vi "DAISY_slow_control_2_15.vi"() -> ()   [LabVIEW 2018]
uses:
  4623b864-5764-45c6-9cb2-3e18237880ca.vi
  fa57f61f-0bb9-49ac-92eb-fcb40add4dbb.vi
  <vilib>/DAQmx/read.llb/DAQmx Read (Analog 1D DBL NChan 1Samp).vi
  ffb0d1b3-ef19-4e2e-b36e-7277177ef4b3.vi
  9a1acc8a-69db-4048-9e4c-bb07d66d2422.vi
  <vilib>/DAQmx/create/channels.llb/DAQmx Create Channel (AI-Voltage-Basic).vi
  <vilib>/DAQmx/create/channels.llb/DAQmx Create Channel (AI-Current-Basic).vi
  <vilib>/DAQmx/create/channels.llb/DAQmx Create Channel (AI-Temperature-RTD).vi
  <vilib>/DAQmx/miscellaneous.llb/DAQmx Fill In Error Info.vi
  <vilib>/Utility/file.llb/Read Delimited Spreadsheet (string).vi
  <instrlib>/Lake Shore 335/Lake Shore 335.lvlib
  <instrlib>/CAEN PSM/CAEN PSM.lvlib
  <resource>/objmgr/daqmx.rc
panel:
  out "Heater":dbl
  out "Coldhead":dbl
  out "Cycle number":i32
  out "Alarm state":bool
  out "Timestamp last \nmeasured (UPS)":timestamp
  out "Auto-clear":bool
  in  "Auto-clear data?":bool
  in  "Clear data":bool
  in  "Clear data every N cycles":dbl=1000000.0
  in  "N samples":i32=30
  out "Average Flow (SLPM)":dbl caption="Flow (SLPM)"
  out "CAEN Ch. Names":string[](array[string])
  in  "Cycles to execute":dbl=5.0 format="%#_13g"
  out "Detector Pressure":dbl
  in  "N samples":i32=20
  in  "Allows tabs on \nfront panel":T1(tab)
  in  "Anode ch.":enum16{"1", "2", "3", "4"}(ring)=enum."3"
  in  "CAEN unit selector":enum16{"CAEN 1", "CAEN 2"}(ring)
  in  "Multipliers":dbl[](array[numeric])=[1.0, 1.0, 1.0, 1.0, 1.0, 1.0, 1.0, 1.0]
  in  "Offsets\nsubtracted":dbl[](array[numeric])=[0.0, 0.0, 0.0, 0.0, 0.0, 0.0, 0.0, 0.0]
  in  "Channel Names (9207, ai8:15)":string[](array[string])=["i0", "i1", "i2", "i3", "i4", "i5", "i6", "i7"] caption="\"Other\""
  in  "Flow meter input:":u16(ring)=3 items=["v0", "v1", "v2", "v3", "v4", "v5", "v6", "v7"]
  in  "Detector pressure input:":u16(ring) items=["v0", "v1", "v2", "v3", "v4", "v5", "v6", "v7"]
  in  "Channel Names (9207, ai0:7)":string[](array[string])=["v0", "v1", "v2", "v3", "v4", "v5", "v6", "v7"] caption="\"Other\""
  in  "Multipliers":dbl[](array[numeric])=[1.0, 1.0, 1.0, 1.0, 1.0, 1.0, 1.0, 1.0]
  in  "Offsets\nsubtracted":dbl[](array[numeric])=[0.0, 0.0, 0.0, 0.0, 0.0, 0.0, 0.0, 0.0]
  in  "Voltage channels":tag[](array[tag])=["9207/ai0", "9207/ai1", "9207/ai2", "9207/ai3", "9207/ai4", "9207/ai5", "9207/ai6", "9207/ai7"]
  in  "COM-port CAEN":refnum<visa-resource-name>
  in  "Run lakeshore?":bool
  in  "ID Query":bool
  in  "COM-port LakeShore":refnum<visa-resource-name>
  in  "PID settings":cluster{"P":dbl, "I":dbl, "D":dbl}={"P"=50.0, "I"=20.0, "D"=120.0}
  in  "Heater range":u16(ring) items=["Off", "Low (On)", "Medium", "High"]
  in  "Current channels":tag[](array[tag])=["9207/ai8", "9207/ai9", "9207/ai10", "9207/ai11", "9207/ai12", "9207/ai13", "9207/ai14", "9207/ai15"]
  in  "Channel Names (CAEN)":string[](array[string])=["PMT 1", "PMT 2", "Anode", "Cathode", "Top gate", "Bottom gate", "Other 1", "Other 2"]
  in  "RTD Type":i32(ring)=10071 items=["Pt3750"=12481, "Pt3851"=10071, "Pt3911"=12482, "Pt3916"=10069, "Pt3920"=10053, "Pt3928"=12483, "Custom"=10137]
  in  "Module 1 channels (slot 1)":tag[](array[tag])=["cDAQ2Mod2/ai0", "cDAQ2Mod2/ai1", "cDAQ2Mod2/ai2", "cDAQ2Mod2/ai3", "cDAQ2Mod2/ai4", "cDAQ2Mod2/ai5", "cDAQ2Mod2/ai6", "cDAQ2Mod2/ai7"]
  in  "Resistance Configuration":i32(ring)=3 items=["3-Wire"=3, "4-Wire"=4]
  in  "R (T = 0°C):":dbl=100.0 format="%_4g"
  in  "B":dbl
  in  "A":dbl
  in  "C":dbl
  in  "Module 2 channels (slot 2)":tag[](array[tag])=["cDAQ2Mod3/ai0", "cDAQ2Mod3/ai1", "cDAQ2Mod3/ai2", "cDAQ2Mod3/ai3", "cDAQ2Mod3/ai4", "cDAQ2Mod3/ai5", "cDAQ2Mod3/ai6", "cDAQ2Mod3/ai7"]
  in  "Shut off heater \nif Alarm is active":bool=TRUE
  in  "Re-save headers":bool
  in  "Resistance Configuration":i32(ring)=3 items=["3-Wire"=3, "4-Wire"=4]
  in  "Module 3 channels":tag[](array[tag])
  in  "RTD Type":i32(ring)=12481 items=["Pt3750"=12481, "Pt3851"=10071, "Pt3911"=12482, "Pt3916"=10069, "Pt3920"=10053, "Pt3928"=12483, "Custom"=10137]
  in  "R (T = 0°C)":dbl=1000.0 format="%0.1f"
  in  "Ignore Initialization Errors":bool=TRUE caption="Ignore init. errors?"
  out "Started up?":bool
  out "heater":i32
  in  "Setpoint (°C)":dbl=-100.0 format="%.1f"
  in  "Kill all channels":bool
  in  "Scale.Range:Minimum 8":dbl
  in  "Scale.Range:Maximum 8":dbl=4000.0
  in  "Scale.Range:Minimum 7":dbl
  in  "Scale.Range:Maximum 7":dbl=4000.0
  in  "Scale.Range:Minimum 6":dbl=-3000.0
  in  "Scale.Range:Maximum 6":dbl
  in  "Scale.Range:Minimum 5":dbl
  in  "Scale.Range:Maximum 5":dbl=3000.0
  in  "Scale.Range:Minimum 4":dbl=-5000.0
  in  "Scale.Range:Maximum 4":dbl
  in  "Scale.Range:Maximum 3":dbl=4000.0
  in  "Scale.Range:Minimum 3":dbl
  in  "Scale.Range:Maximum 2":dbl=1000.0
  in  "Scale.Range:Minimum 2":dbl
  out "CAEN 1.1":dbl(knob) scale=0.0..1000.0
  out "CAEN 1.1":string
  in  "Scale.Range:Maximum":dbl=1000.0
  in  "Scale.Range:Minimum":dbl
  out "CAEN 2.3 2":string
  out "CAEN 2.2 2":string
  out "Channel Names":string[](array[string])
  out "CAEN 2.3":dbl(knob) scale=0.0..4000.0
  out "CAEN 2.2":dbl(knob) scale=0.0..4000.0
  out "CAEN 2.1":string
  out "CAEN 2.0":string
  out "CAEN 1.3":string
  out "CAEN 1.2":string
  out "CAEN 1.0":string
  out "Channel Names":string[](array[string])
  in  "Set to zero (ramp down)":bool
  out "CAEN 2.1":dbl(knob) scale=0.0..-3000.0
  out "CAEN 2.0":dbl(knob) scale=0.0..3000.0
  in  "Apply Voltage":bool
  in  "VSet (V)":dbl[](array[numeric])
  in  "IMax (uA)":dbl[](array[numeric])
  in  "VMax (V)":dbl[](array[numeric])
  out "CAEN 1.3":dbl(knob) scale=0.0..-5000.0
  out "CAEN 1.2":dbl(knob) scale=0.0..4000.0
  out "CAEN 1.0":dbl(knob) scale=0.0..1000.0
  out "Vmon (V)":dbl[](array[numeric])
  out "IMon (uA)":dbl[](array[numeric])
  in  "Reset anode\nperiodically?":bool
  in  "Kill every Y minutes":i32=10
  in  "Keep off for X seconds":i32=10
  out "?":bool
  out "Killed":bool
  out "Restarted":bool
  out "Anode timers":timestamp[](array[timestamp])
  out "Seconds until \nanode autokill":dbl format="%.2g"
  out "Seconds until \nanode reset":dbl format="%.2g"
  in  "Temperature channel selector":u16(ring) items=["0"=0, "1"=1, "2"=2, "3"=3, "4"=4, "5"=5, "6"=6, "7"=7, "Average"=666]
  out "Heater power (%)":cluster{timestamp[], dbl[]}[](graph)
  out "Flow (SLPM)":cluster{timestamp[], dbl[]}[](graph)
  out "9207 (ai 0:7, Volts)":cluster{timestamp[], dbl[]}[](graph)
  out "Phase Diagram":cluster{"X":dbl, "Y":dbl}[](graph)
  out "Setup Temperature (9216 0:15, °C)":cluster{timestamp[], dbl[]}[](graph)
  out "LakeShore readings":dbl[](array[numeric])
  out "Low Temperature (9226 0:7 and LakeShore A;B, °C)":cluster{timestamp[], dbl[]}[](graph)
  in  "Reset?":bool
  out "Integrated Flow (SL)":dbl
  in  "Pause?":bool
  in  "\"Sound\" alarm":bool
  in  "Sound alarm\nFrequency (Hz)":dbl=1260.0
  in  "Send status email now":bool
  out "Email error":i32
  out "source":string
  in  "Number of Bonus lines":i32=1
  out "Names (optional)":string[](array[string])
  in  "Send daily email?":bool=TRUE
  in  "Phone numbers":string[](array[string])
  out "Alarm (or test) message":string
  in  "Alarm\nMaster switch":bool
  in  "Repeat Alarm SMS\nevery N minutes":dbl=15.0
  in  "Test alarm":bool
  out "Warning":bool
  in  "UPS":bool
  in  "UPS Voltage \nLower Threshold":dbl=220.0
  out "NI mod 2&3 status":bool
  in  "NI mod 2&3":bool
  in  "NI mod 1":bool
  in  "CAEN 2":bool
  in  "CAEN 1":bool
  in  "LakeShore":bool
  out "Det. P. warning":bool
  out "Boolean 6":bool
  out "Boolean 5":bool
  out "Boolean 4":bool
  out "Boolean 3":bool
  out "Boolean 2":bool
  out "Boolean":bool
  in  "T 6":bool
  in  "T 5":bool
  in  "T 4":bool
  in  "T 3":bool
  in  "T 2":bool
  in  "T 1":bool
  in  "Detector Pressure":bool
  in  "Overpressure threshold":dbl
  in  "Underpressure threshold":dbl
  out "Comm. status":bool
  in  "High Temp threshold":dbl format="%#_13g"
  in  "Low Temp threshold":dbl format="%#_13g"
  out "LakeShore status":bool
  out "NI mod1 (P) status":bool
  out "CAEN 1 status":bool
  out "CAEN 2 status":bool
  out "Initialization status":bool
  out "Minimum input voltage measured":dbl
  out "Alarm active 2":bool
  out "SMS error":string
  out "Status email preview":string
  in  "Send status email at time:":string="14:00"
  in  "Email Addresses":string[](array[string])
  in  "return address":string="xamsups@gmail.com"
  out "NI 9226":errorcluster
  in  "HV Channel status":string="Click the button to request the latest High Voltage channel status.\nView another channel with the arrows, or typing 0 through 3."
  out "CAEN 1":T2(array[cluster])
  out "CAEN 2":T2(array[cluster])
  in  "Query HV status":bool
  in  "LabVIEW error code":string="Google this"
  in  "String 7":string="A checkmark means \"No error\" and false. A red X means an error occurred"
  out "\"status\"":bool
  in  "\"source\"":string="This may show two things: the latest executed VI in the task chain, in reverse order, or: which VI produced an error, with a short description. If the error can't easily be resolved, google the code."
  out "NI 9216 x2":errorcluster
  out "CAEN 1":errorcluster
  out "CAEN 2":errorcluster
  out "Lakeshore":errorcluster
  out "NI 9207":errorcluster
  out "Temp A":dbl
  out "Temp B":dbl
  in  "Temperature Channel Selector":u16(ring) items=["0", "1", "2", "3", "4", "5", "6", "7"]
  out "Historical Large Phase Diagram":cluster{dbl[], dbl[]}[](graph)
  out "Large Phase Diagram":cluster{"X":dbl, "Y":dbl}[](graph)
  in  "Temperature Channel Selector":u16(ring) items=["0"=0, "1"=1, "2"=2, "3"=3, "4"=4, "5"=5, "6"=6, "7"=7, "Average"=666]
  out "PT1000 data":dbl[](array[numeric]) format="%0.2f"
  out "9207 (V; A) Converted":dbl[](array[numeric])
  out "9216 #1 (°C)":dbl[](array[numeric])
  out "9216 #2 (°C)":dbl[](array[numeric])
  out "Raw readouts (V, mA)":dbl[](array[numeric]) format="%0.2f"
  out "Det.P input #":i32
  out "Flow input #":i32
  out "PT100 data":dbl[](array[numeric]) format="%0.2f"
  out "9207 (ai 8:15, Amperes)":cluster{timestamp[], dbl[]}[](graph)
  in  "Kill voltage":bool
  in  "stop":bool
  out "Voltages":dbl[](array[numeric])
  out "TOBA appended":dbl[][](array[numeric])
  in  "Read T every N cycles":i32=2
  out "Time until next cycle":dbl format="%.3g"
  in  "Time per cycle (s)":i32=2 caption="Time Target (s)"
  # "<- Proof of concept for New/Old T + New P"
  # "Remove ^this^ array, just for testing and takes up lots of resources"
  # "Moving averages"
  # "CAEN settings"
  # "NI 9216 Temperature settings"
  # "NI 9207 Voltage settings"
  # "NI 9207 Current settings"
  # "If RTD type is custom,\nspecify the Callendar-\nVan Dusen parameters"
  # "Anode connected to:"
  # "Channel:"
  # "Lakeshore settings"
  # "NI 9226 Temperature settings"
  # "Miscellaneous"
  # "Gain (P) (XX.X)"
  # "Reset (I) (XX.X)"
  # "Rate (D) (X.X%)"
  # "Data"
  # "Scale:"
  # "to"
  # "to"
  # "Scale:"
  # "Time of last reset"
  # "Time of last reactivation"
  # "to"
  # "Scale:"
  # "to"
  # "Scale:"
  # "Settings"
  # "Scale:"
  # "to"
  # "Scale:"
  # "to"
  # "Scale:"
  # "to"
  # "to"
  # "Scale:"
  # "ADD LAKESHORE TEMPS"
  # "Alarm indicators and arms"
  # "Detector Thresholds"
  # "Daily status email"
  # "SMS and sound alarm"
  # "Alarm conditions"
  # "Temperature channels:"
  # "Uninterruptable Power Supply"
  # "Task information"
  # "High Voltage channel status"
  # "Error info example"
  # "Channel"
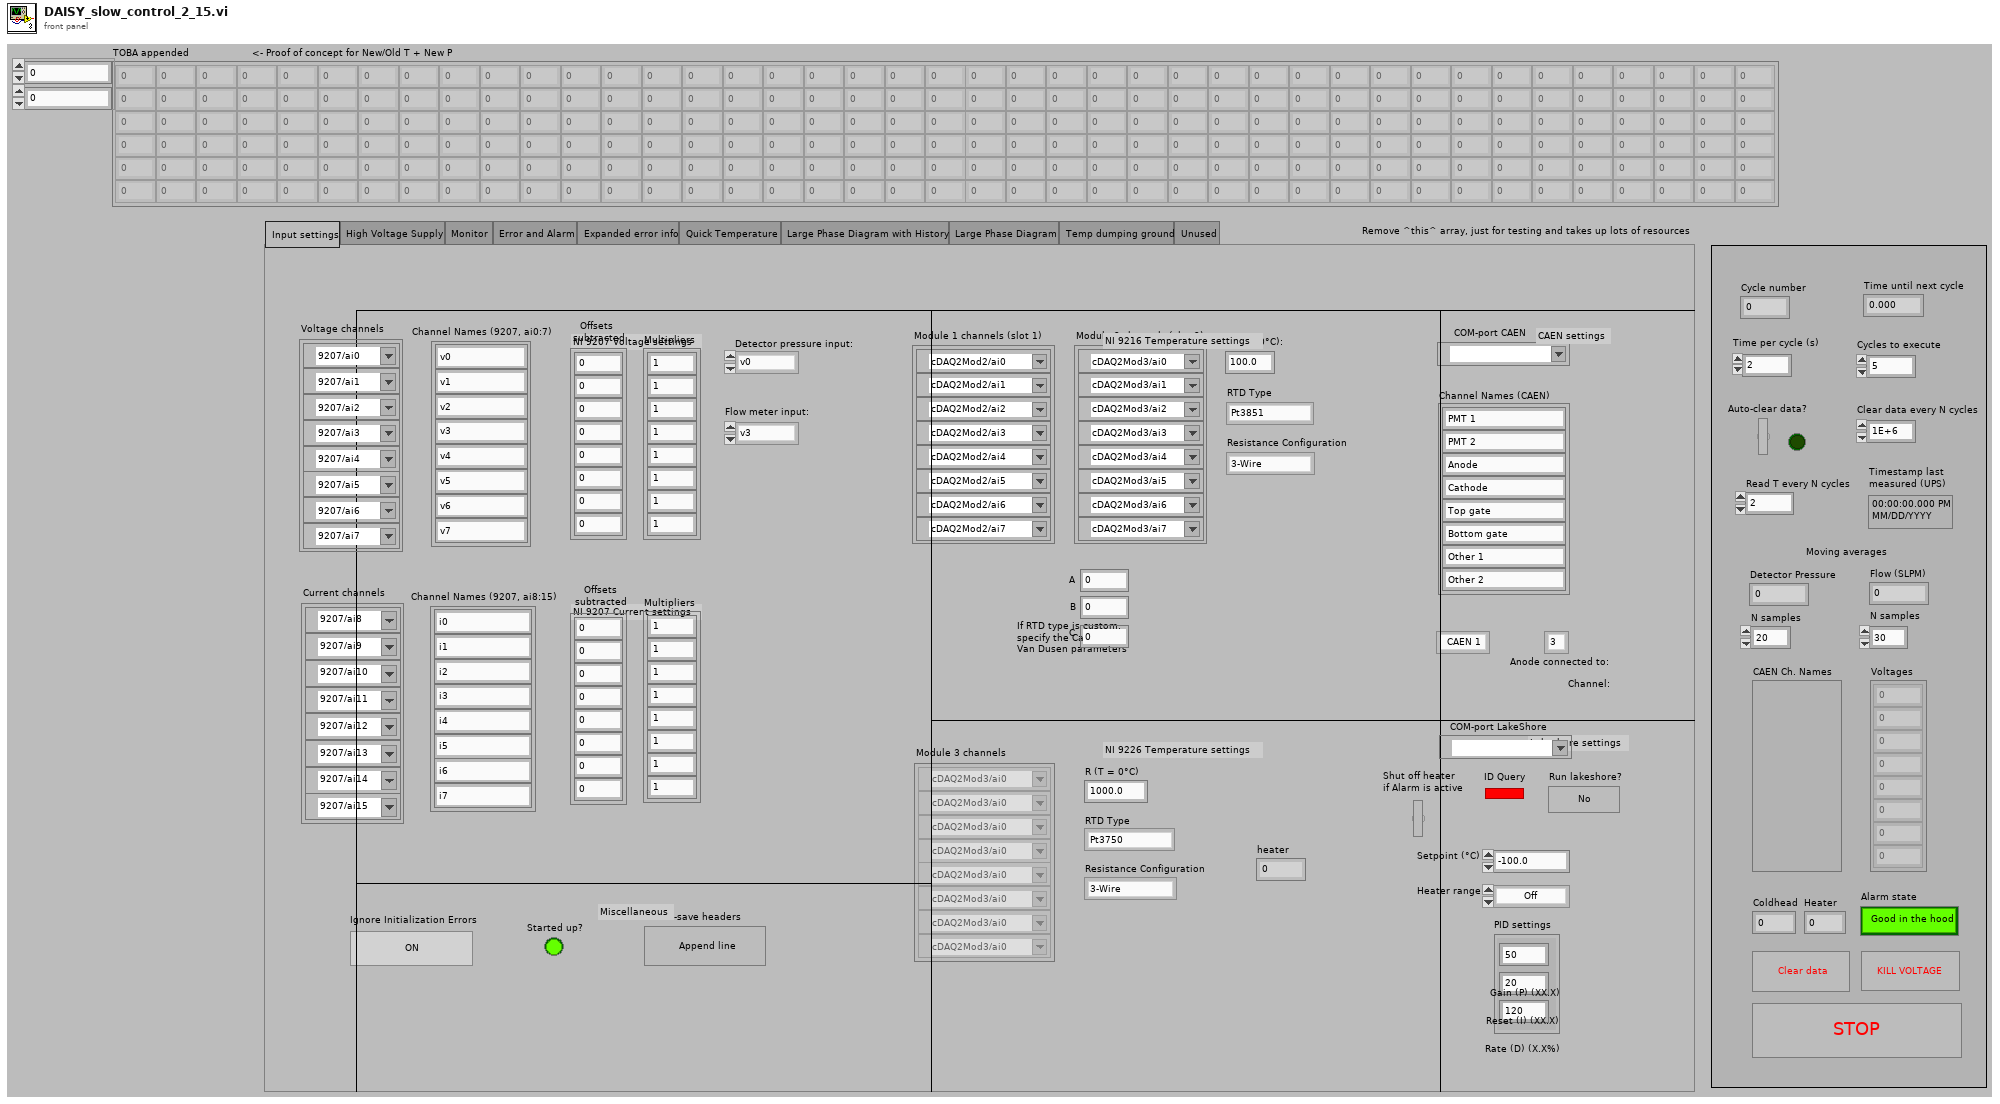
[diagram p1: front panel]
types:
  T1 = enum32{"Input settings", "High Voltage Supply", "Monitor", "Error and Alarm", "Expanded error info", "Quick Temperature", "Large Phase Diagram with History", "Large Phase Diagram", "Temp dumping ground", "Unused"}
  T2 = cluster{"ON":bool, "RUP":bool, "RDW":bool, "OVC":bool, "OVV":bool, "UNV":bool, "MAXV":bool, "TRIP":bool, "OVP":bool, "OVT":bool, "DIS":bool, "KILL":bool, "ILK":bool, "NOCAL":bool}[]
  T3 = cluster{"Baud Rate":u32, "Parity":u16, "Data Bits":u16, "Stop Bits":u16, "Flow Control":u16}
  T4 = typedef "CAEN PSM.lvlib/BoardHandle.ctl" = cluster{"VISA resource name":refnum<visa-resource-name>, "Board address":u8, "NChannels":u8}
  T5 = cluster{"task out":refnum<k21>, "error out":errorcluster}
  T6 = cluster{"VISA resource name out":refnum<visa-resource-name>, "error out":errorcluster}
  T7 = cluster{"VISA resource name":refnum<visa-resource-name>, "Board address":u8, "NChannels":u8}[]
  T8 = cluster{"VISA resource name":refnum<visa-resource-name>, "Board address":u8, "NChannels":u8}
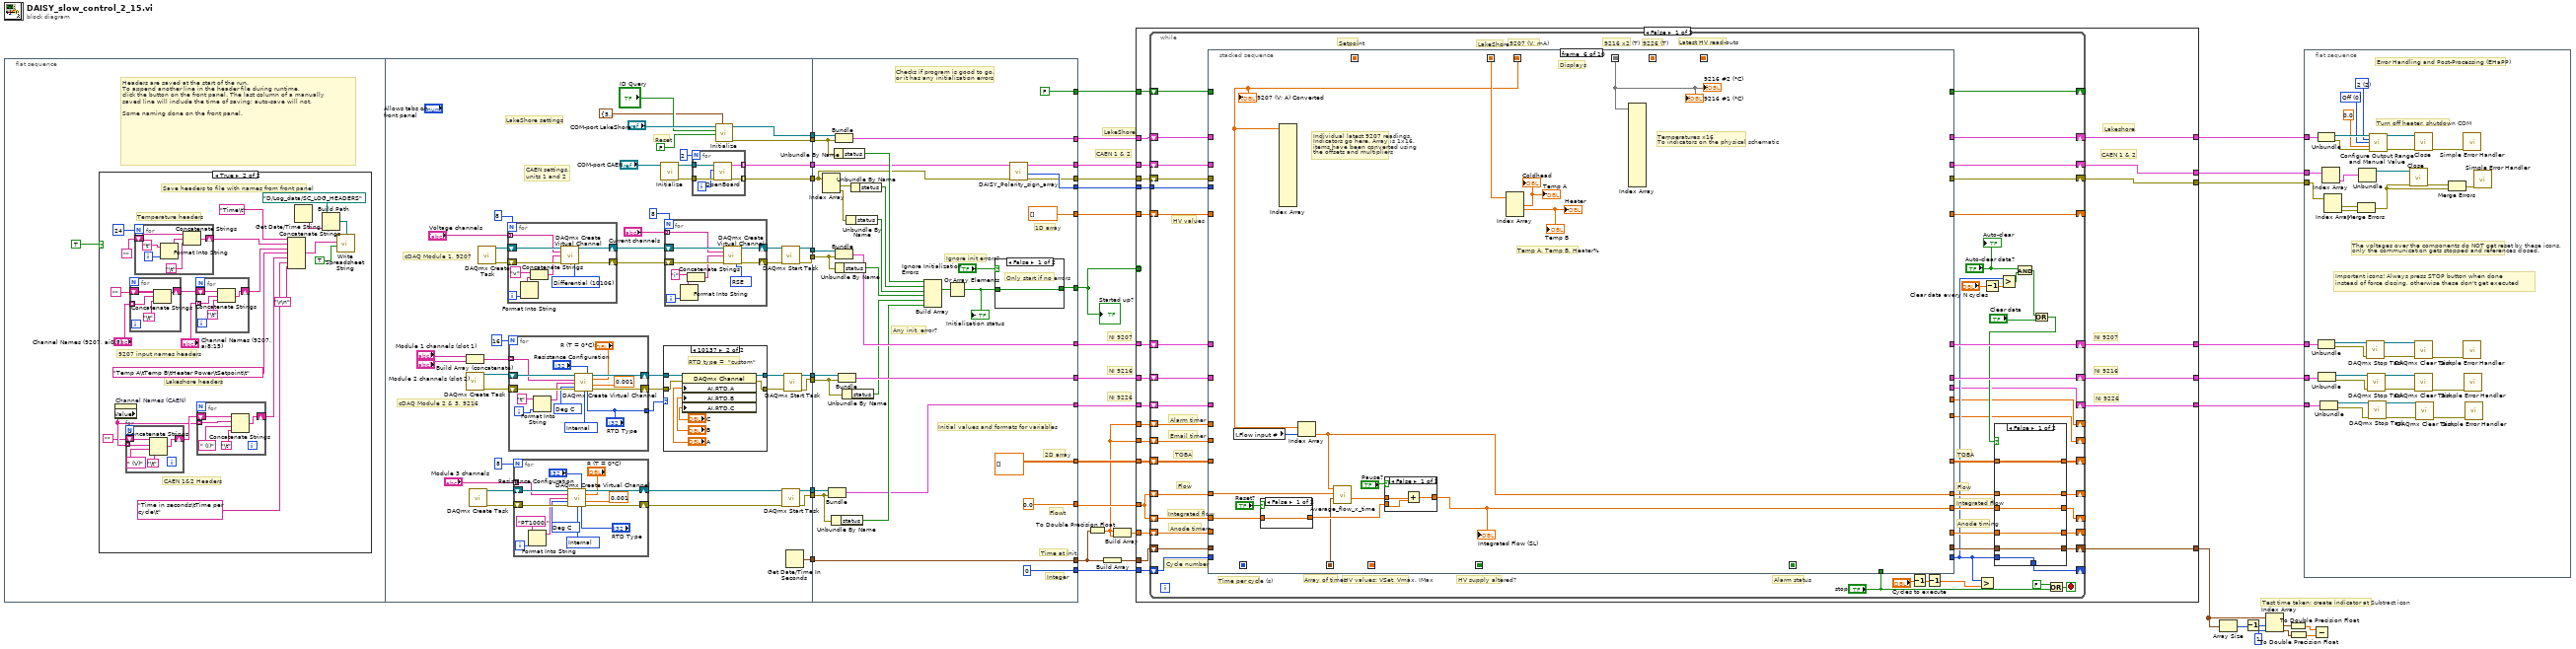
[diagram p0: block diagram]
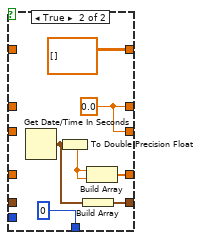
[diagram p2: hidden frame]
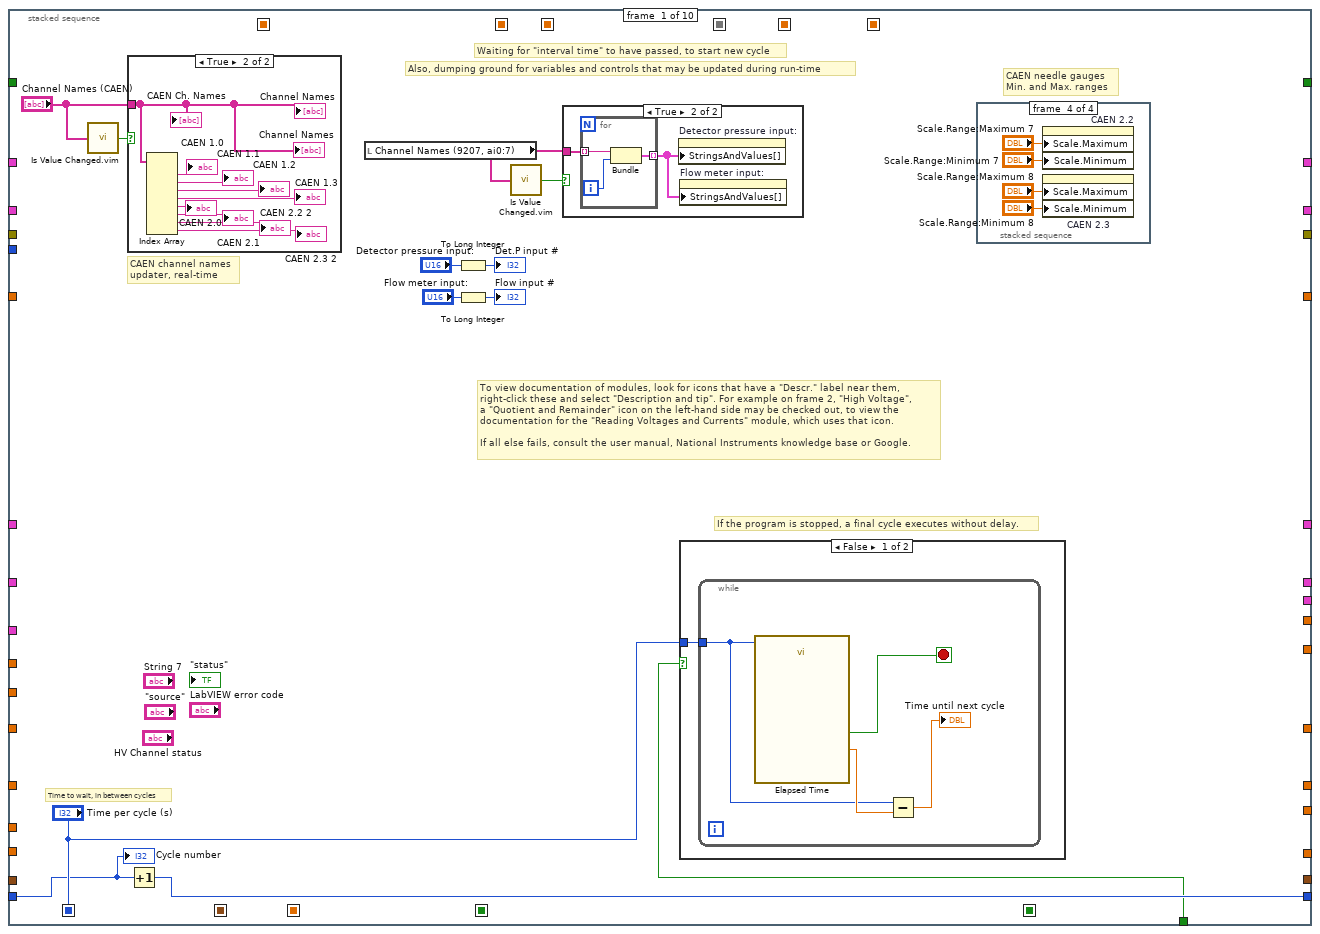
[diagram p3: hidden frame]
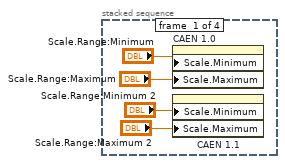
[diagram p6: hidden frame]
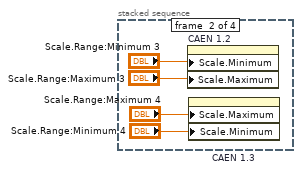
[diagram p7: hidden frame]
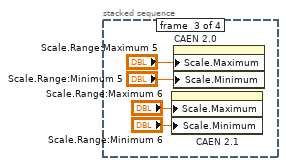
[diagram p8: hidden frame]
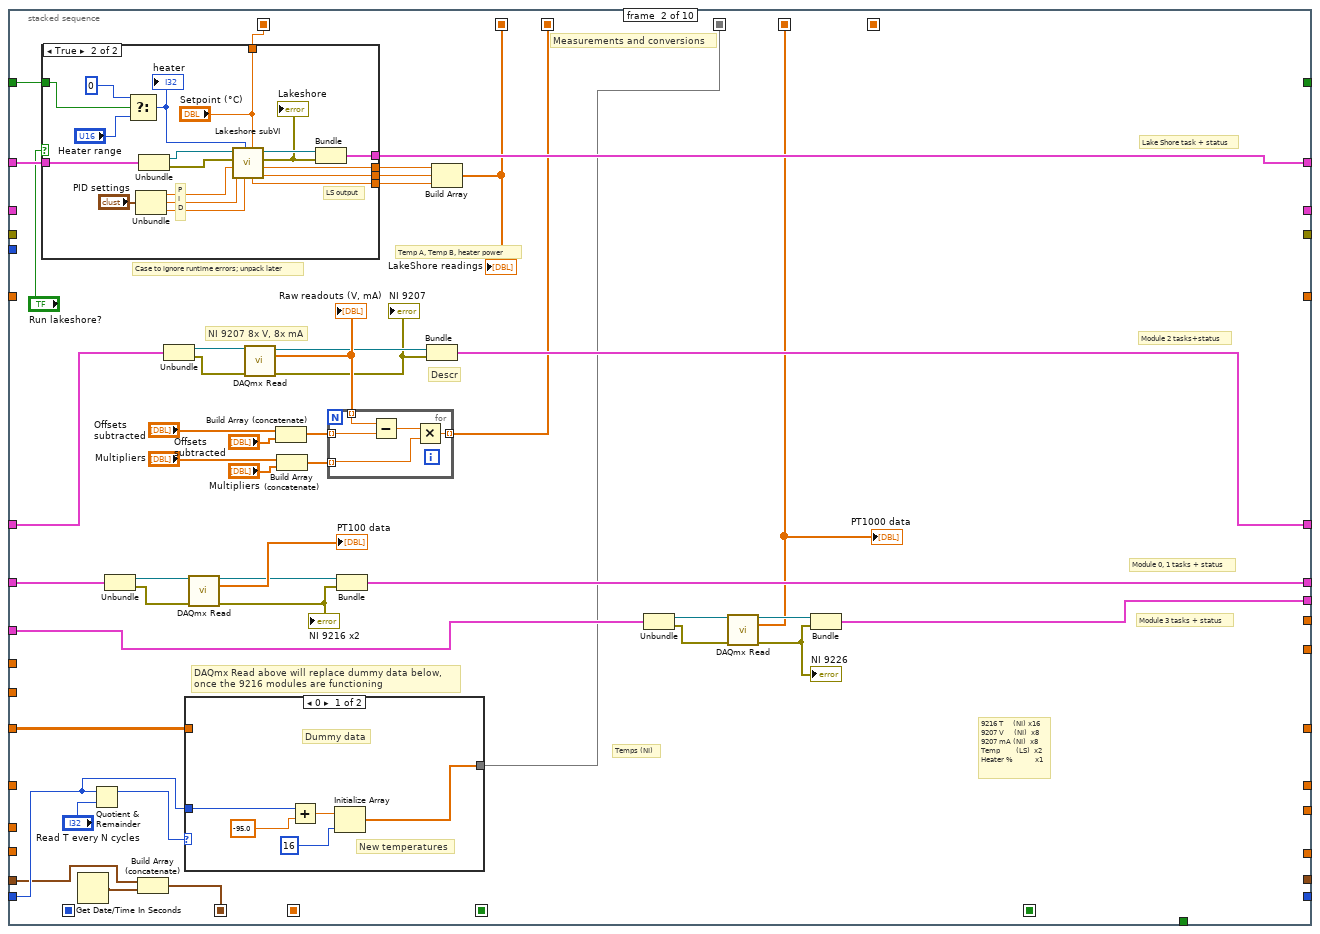
[diagram p10: hidden frame]
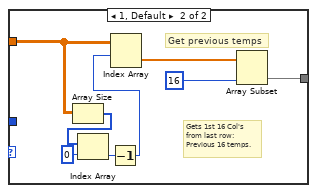
[diagram p11: hidden frame]
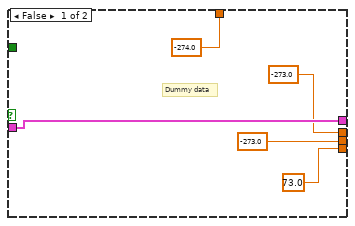
[diagram p12: hidden frame]
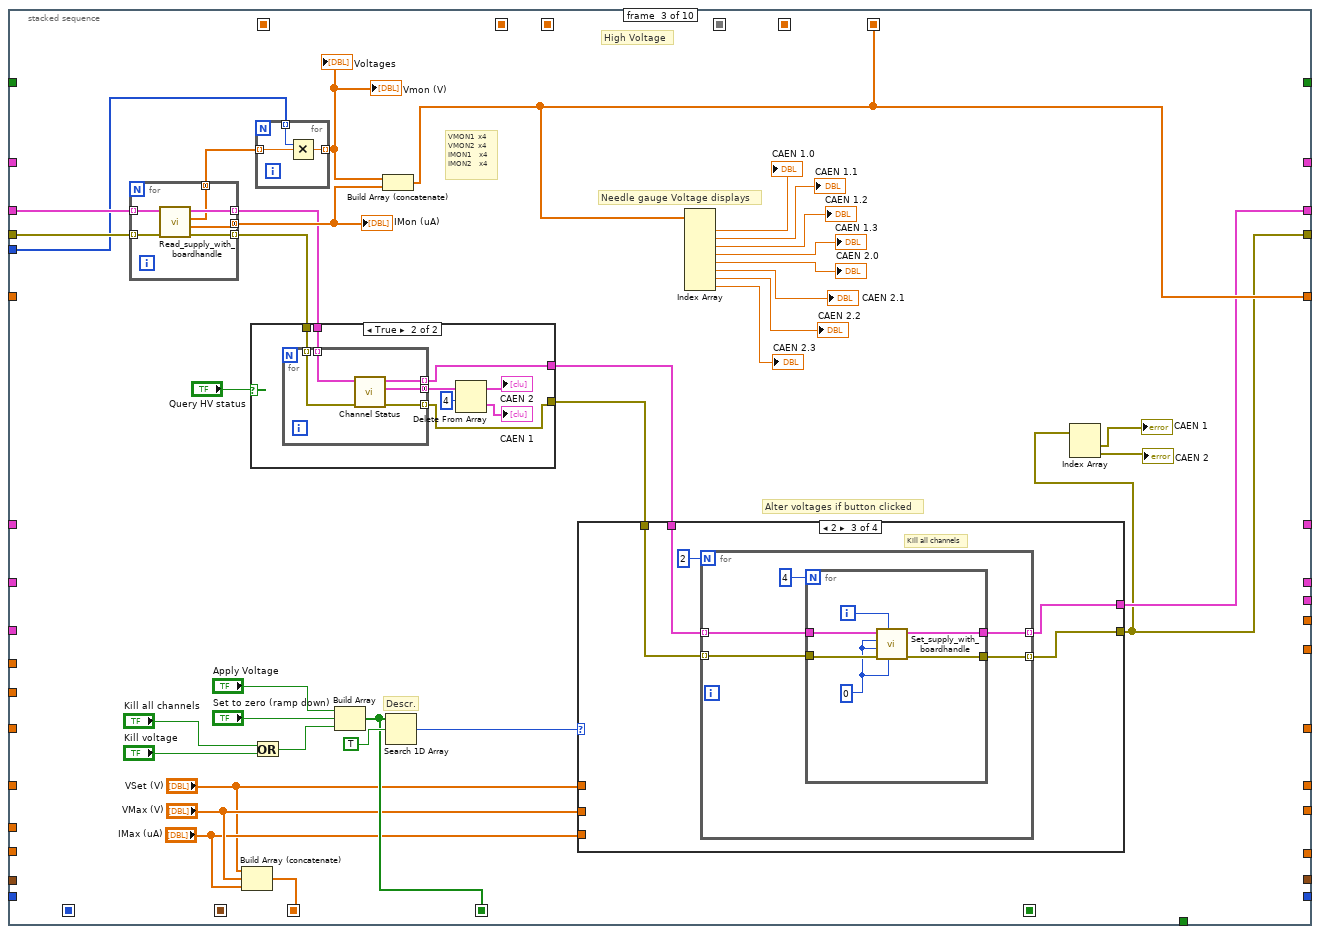
[diagram p13: hidden frame]
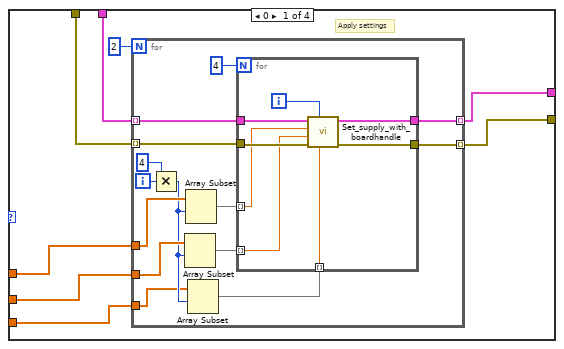
[diagram p14: hidden frame]
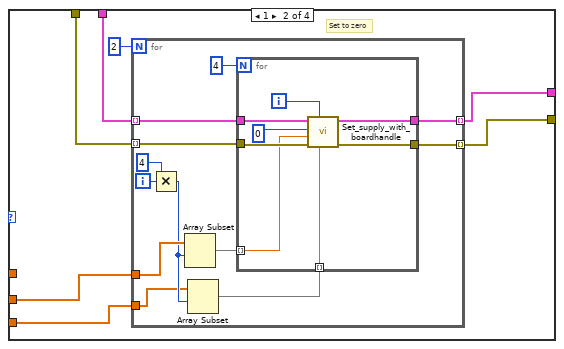
[diagram p15: hidden frame]
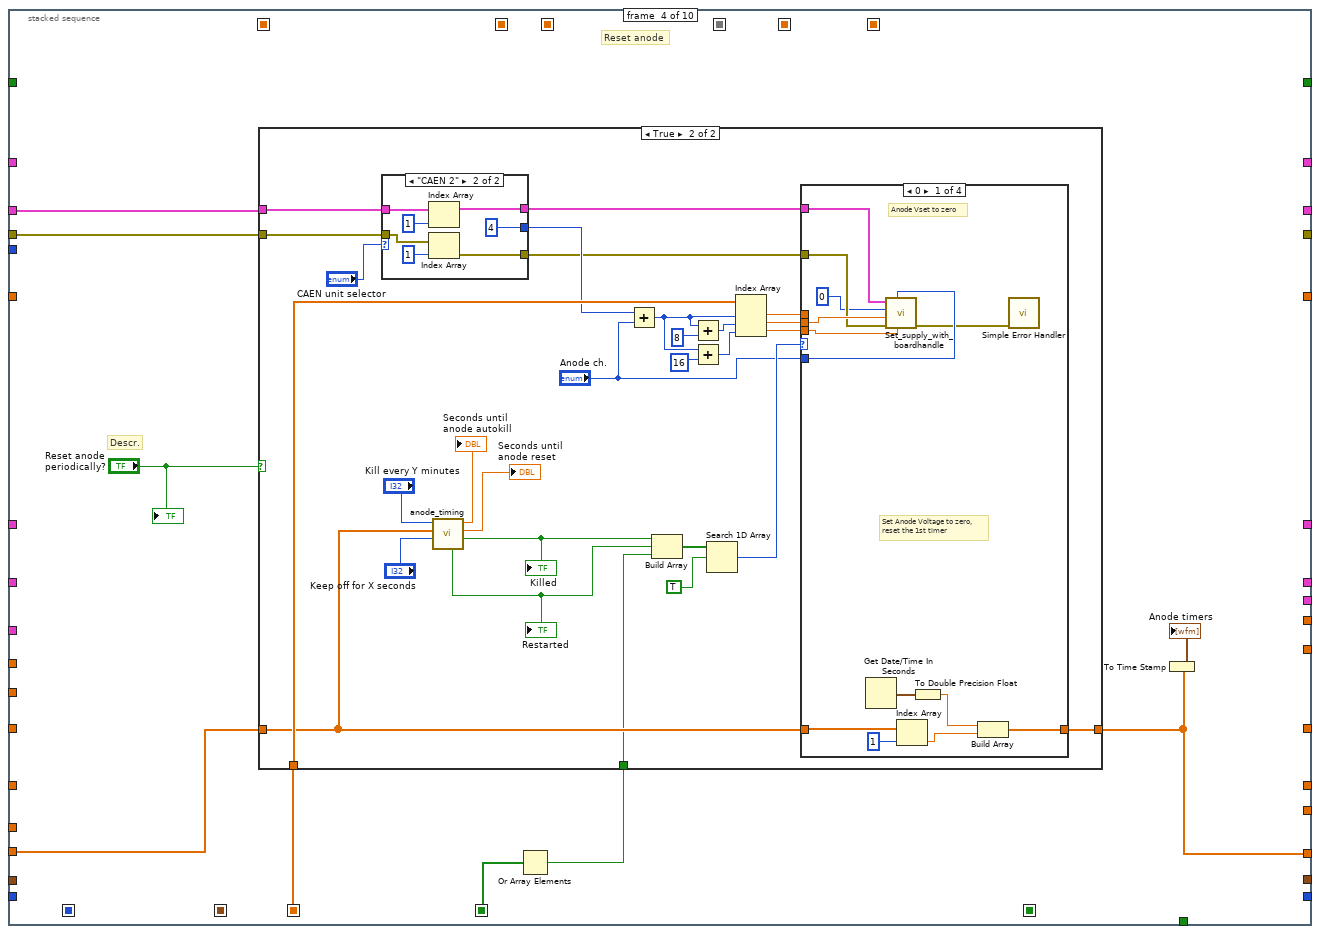
[diagram p18: hidden frame]
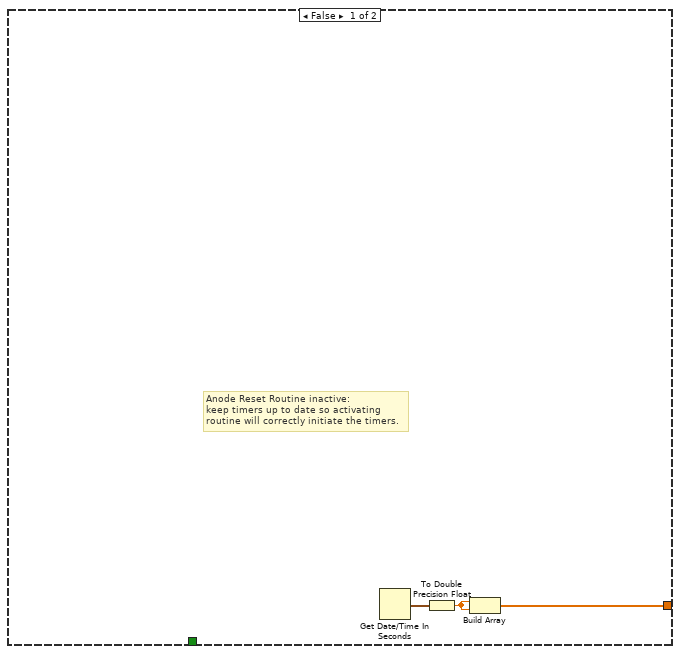
[diagram p19: hidden frame]
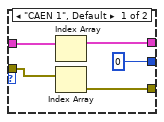
[diagram p20: hidden frame]
diagram:
  # "NI 9226"
  # "NI 9216"
  # "Test time taken: create indicator at Subtract icon"
  # "NI 9207"
  # "CAEN 1 & 2"
  # "LakeShore"
  n1 = flat-sequence {
    tunnel: [w131] -> w42
    tunnel: [w130] -> w41
    tunnel: [w127] -> w40
    tunnel: [w115] -> w39
    tunnel: [w126] -> w35
    tunnel: [w116] -> w21
    tunnel: [w110] -> w14
    tunnel: [w109] -> w13
    tunnel: [w95] -> w9
    tunnel: [w94] -> w8
    tunnel: [w90] -> w4
    tunnel: w42 -> [w228]
    tunnel: w41 -> [w227]
    tunnel: w40 -> [w200]
    tunnel: w39 -> [w220]
    tunnel: [w229] -> w27
    tunnel: [0.0] -> w26
    tunnel: [dbl[] []] -> w38
    tunnel: [dbl[][] []] -> w15
    tunnel: [0] -> w37
    tunnel: [w226] -> w36
    tunnel: [w225] -> w25
    tunnel: w35 -> [w225]
    tunnel: [FALSE] -> w22
    tunnel: w21 -> [w221]
    tunnel: [w219] -> w20
    tunnel: w14 -> [w212]
    tunnel: w13 -> [w211]
    tunnel: [w210] -> w12
    tunnel: w9 -> [w207]
    tunnel: w8 -> [w206]
    tunnel: [w204] -> w7
    tunnel: [w199] -> w5
    tunnel: w4 -> [w201]
    tunnel: [w198] -> w3
    tunnel: [w197] -> w2
    frame #0 {
      # "Headers are saved at the start of the run.\nTo append another line in the header file during runtime,\nclick the button on the front panel. The last column of a manually\nsaved line will include the time of saving; auto-save will not.\n\nSome naming done on the front panel."
      n2 = case shown="True" TRUE {
        frame False {
        }
        frame True {
          # "CAEN 1&2 Headers"
          # "Lakeshore headers"
          # "9207 input names headers"
          # "Temperature headers"
          # "Save headers to file with names from front panel"
          n3 = property on="Channel Names (CAEN)" class="Arr (strict)"() -> ("Value"=w49:string[])  [unwired: 2 in, 2 out]
          n4 = for {
            tunnel: w49 -> [w73] mode=indexing
            shift-right: [w71] -> w50
            shift-left: "" -> [w70]
            n5 = Concatenate Strings(w70, w73, " (V)", "\t") -> (w71:string)
          }
          n6 = for {
            shift-right: [w81] -> w53
            shift-left: "" -> [w82]
            tunnel: "Channel Names (9207, ai0:7)" -> [w79] mode=indexing
            n7 = Concatenate Strings(w82, w79, "\t") -> (w81:string)
          }
          n8 = for {
            N: 24 -> [_]
            shift-right: [w83] -> w56
            shift-left: "" -> [w84]
            i -> [w88]
            n9 = Format Into String(initial string="t", w88) -> (resulting string=w86:string)  [unwired: 2 in, 1 out]
            n10 = Concatenate Strings(w84, w86, "\t") -> (w83:string)
          }
          n11 = for {
            shift-right: [w76] -> w52
            shift-left: w53 -> [w78]
            tunnel: "Channel Names (9207, ai8:15)" -> [w75] mode=indexing
            n12 = Concatenate Strings(w78, w75, "\t") -> (w76:string)
          }
          n13 = for {
            shift-right: [w66] -> w48
            shift-left: w50 -> [w67]
            tunnel: w49 -> [w65] mode=indexing
            n14 = Concatenate Strings(w67, w65, " (I)", "\t") -> (w66:string)
          }
          n15 = Concatenate Strings("Time\t", w56, w52, "Temp A\tTemp B\tHeater Power\tSetpoint\t", w48, "Time in seconds\tTime per cycle\t", "\r\n") -> (w55:string)
          n16 = Get Date/Time String() -> (date string=w59:string)  [unwired: 3 in, 1 out]
          n17 = Build Path(base path=path "D:/Log_data/SC_LOG_HEADERS" ("file path (dialog if empty)"), name or relative path=w59) -> (appended path=w60:path)
          n18 = call <vilib>:"Write Spreadsheet String.vi"("append to file? (new file:F)"=TRUE, "spreadsheet string"=w55, "file path (dialog if empty)"=w60) -> ()  [unwired: 7 in, 2 out]
        }
      }
    }
    frame #1 {
      # "cDAQ Module 2 & 3, 9216"
      # "cDAQ Module 1, 9207"
      # "CAEN settings,\nunits 1 and 2"
      # "Reset"
      # "LakeShore settings"
      n19 = call <vilib>:"DAQmx Create Task.vi"() -> ("task out"=w92:refnum<k21>, "error out"=w111:errorcluster)  [unwired: 14 in]
      n20 = Build Array (concatenate)("Module 1 channels (slot 1)", "Module 2 channels (slot 2)") -> (w106:tag[])
      n21 = call <vilib>:"DAQmx Create Task.vi"() -> ("task out"=w100:refnum<k21>, "error out"=w99:errorcluster)  [unwired: 14 in]
      n22 = call <vilib>:"DAQmx Create Task.vi"() -> ("task out"=w123:refnum<k21>, "error out"=w122:errorcluster)  [unwired: 14 in]
      n23 = for {
        N: 8 -> [_]
        shift-right: [w192] -> w120
        shift-left: w123 -> [w191]
        shift-right: [w193] -> w119
        shift-left: w122 -> [w189]
        tunnel: "Voltage channels" -> [w190] mode=indexing
        i -> [w195]
        w187 = 10106 items=["Default"=-1, "RSE"=10083, "NRSE"=10078, "Differential"=10106, "Pseudodifferential"=12529] ("input terminal configuration")
        n24 = Format Into String(w195) -> (resulting string=w194:string)  [unwired: 3 in, 1 out]
        n25 = Concatenate Strings("v" ("string"), w194) -> (w188:string)
        n26 = call-poly <vilib>:"DAQmx Create Virtual Channel.vi"("task in"=w191, "input terminal configuration"=w187, "physical channels"=w190, "name to assign"=w188, "error in"=w189) -> ("task out"=w192:refnum<k21>, "error out"=w193:errorcluster)  [unwired: 9 in]
      }
      n27 = for {
        N: 16 -> [_]
        shift-right: [w173] -> w91
        shift-left: w92 -> [w176]
        shift-right: [w174] -> w105
        shift-left: w111 -> [w175]
        tunnel: w106 -> [w172] mode=indexing
        tunnel: ["RTD Type"] -> w102
        i -> [w170]
        w168 = 10200 items=["Internal"=10200, "External"=10167, "None"=10230] ("Current Excitation Source")
        w167 = 10143 items=["Deg C"=10143, "Deg F"=10144, "Kelvins"=10325, "Deg R"=10145, "From Custom Scale"=10065] ("units")
        n28 = Format Into String(initial string="t", w170) -> (resulting string=w169:string)  [unwired: 2 in, 1 out]
        n29 = call-poly <vilib>:"DAQmx Create Virtual Channel.vi"("task in"=w176, "resistance configuration"="Resistance Configuration", "physical channels"=w172, "r0"="R (T = 0°C):", "name to assign"=w169, "units"=w167, "current excitation value"=0.001, "error in"=w175, "current excitation source"=w168, "rtd type"="RTD Type") -> ("task out"=w173:refnum<k21>, "error out"=w174:errorcluster)  [unwired: 4 in]
      }
      n30 = for {
        N: 8 -> [_]
        shift-right: [w151] -> w97
        shift-left: w100 -> [w150]
        shift-right: [w152] -> w96
        shift-left: w99 -> [w153]
        tunnel: "Module 3 channels" -> [w148] mode=indexing
        i -> [w146]
        w142 = 10200 items=["Internal"=10200, "External"=10167, "None"=10230] ("current excitation source")
        w144 = 10143 items=["Deg C"=10143, "Deg F"=10144, "Kelvins"=10325, "Deg R"=10145, "From Custom Scale"=10065] ("units")
        n31 = Format Into String(initial string="PT1000.", w146) -> (resulting string=w145:string)  [unwired: 2 in, 1 out]
        n32 = call-poly <vilib>:"DAQmx Create Virtual Channel.vi"("task in"=w150, "resistance configuration"="Resistance Configuration", "physical channels"=w148, "r0"="R (T = 0°C)", "name to assign"=w145, "units"=w144, "current excitation value"=0.001, "error in"=w153, "current excitation source"=w142, "rtd type"="RTD Type") -> ("task out"=w151:refnum<k21>, "error out"=w152:errorcluster)  [unwired: 4 in]
      }
      n33 = call <instrlib>:"Initialize.vi"("VISA resource name"="COM-port CAEN") -> ("error out"=w128:errorcluster, "VISA resource name out"=w124:refnum<visa-resource-name>)  [unwired: 9 in]
      n34 = case shown="10137" w102 {
        tunnel: w91 -> [w155 w159]
        tunnel: w105 -> [w154 w158]
        tunnel: [w155 w157] -> w104
        tunnel: [w154 w156] -> w103
        frame 0, Default {
          # "Don't need to specify the A, B, C\nvalues if RTD type is not \"custom\""
        }
        frame 10137 {
          # "RTD type =  \"custom\""
          n35 = property class="DAQmx Channel"(reference=w159, error in=w158, "AI.RTD.A"="A", "AI.RTD.B"="B", "AI.RTD.C"="C") -> (reference out=w157:refnum<k21>, error out=w156:errorcluster)
        }
      }
      n36 = for {
        N: 8 -> [_]
        shift-right: [w178] -> w117
        shift-left: w120 -> [w185]
        shift-right: [w177] -> w118
        shift-left: w119 -> [w184]
        tunnel: "Current channels" -> [w183] mode=indexing
        i -> [w182]
        w186 = 10083 items=["default"=-1, "RSE"=10083, "NRSE"=10078, "Differential"=10106, "Pseudodifferential"=12529] ("input terminal configuration")
        n37 = Format Into String(w182) -> (resulting string=w180:string)  [unwired: 3 in, 1 out]
        n38 = Concatenate Strings("i", w180) -> (w179:string)
        n39 = call-poly <vilib>:"DAQmx Create Virtual Channel.vi"("task in"=w185, "input terminal configuration"=w186, "physical channels"=w183, "name to assign"=w179, "error in"=w184) -> ("task out"=w178:refnum<k21>, "error out"=w177:errorcluster)  [unwired: 9 in]
      }
      n40 = for {
        N: 2 -> [_]
        tunnel: w124 -> [w137]
        tunnel: [w135] -> w90 mode=indexing
        tunnel: w128 -> [w139]
        tunnel: [w138] -> w127 mode=indexing
        i -> [w136]
        n41 = call <instrlib>:"OpenBoard.vi"("error in (no error)"=w139, "Board Address"=w136, "VISA resource name"=w137) -> ("error out"=w138:errorcluster, "BoardHandle"=w135:T4)  [unwired: 7 in]
      }
      n42 = call <instrlib>:"Initialize.vi"("Serial Configuration"=T3 {"Baud Rate"=57600, "Parity"=1, "Data Bits"=7, "Stop Bits"=10, "Flow Control"=0}, "Reset (True)"=FALSE ("Reset (LakeShore)"), "ID Query (True)"="ID Query", "VISA resource name"="COM-port LakeShore") -> ("error out"=w130:errorcluster, "VISA resource name out"=w131:refnum<visa-resource-name>)  [unwired: 6 in]
      n43 = call <vilib>:"DAQmx Start Task.vi"("task/channels in"=w117, "error in"=w118) -> ("task out"=w116:refnum<k21>, "error out"=w115:errorcluster)  [unwired: 12 in]
      n44 = call <vilib>:"DAQmx Start Task.vi"("task/channels in"=w97, "error in"=w96) -> ("task out"=w95:refnum<k21>, "error out"=w94:errorcluster)  [unwired: 12 in]
      n45 = call <vilib>:"DAQmx Start Task.vi"("task/channels in"=w104, "error in"=w103) -> ("task out"=w110:refnum<k21>, "error out"=w109:errorcluster)  [unwired: 12 in]
      n46 = Get Date/Time In Seconds() -> (seconds since 1Jan1904=w126:timestamp)
    }
    frame #2 {
      # "1D array"
      # "Initial values and formats for variables"
      # "Time at init."
      # "Integer"
      # "2D array"
      # "Flowt"
      # "Checks if program is good to go,\nor it has any initialization errors"
      # "Ignore init errors?"
      # "Any init. error?"
      n47 = Index Array(array=w200) -> (element #1=w203:errorcluster, element #2=w202:errorcluster)  [unwired: 2 in]
      n48 = Bundle("task out"=w207, "error out"=w206) -> (w204:T5)  [unwired: 1 in]
      n49 = Unbundle By Name(w206) -> ("status"=w205:bool)
      n50 = Unbundle By Name(w227) -> ("status"=w213:bool)
      n51 = Bundle("VISA resource name out"=w228, "error out"=w227) -> (w226:T6)  [unwired: 1 in]
      n52 = Unbundle By Name(w220) -> ("status"=w214:bool)
      n53 = Bundle("task out"=w221, "error out"=w220) -> (w219:T5)  [unwired: 1 in]
      n54 = Bundle("task out"=w212, "error out"=w211) -> (w210:T5)  [unwired: 1 in]
      n55 = Unbundle By Name(w211) -> ("status"=w209:bool)
      n56 = Unbundle By Name(w202) -> ("status"=w224:bool)
      n57 = Unbundle By Name(w203) -> ("status"=w230:bool)
      n58 = Build Array(w213, w230, w214, w224, w209, w205) -> (w231:bool[])
      n59 = Or Array Elements(Boolean array=w231) -> (logical OR=w208:bool)
      "Initialization status" <- w208
      n60 = case shown="False" "Ignore Initialization Errors" {
        tunnel: [w232 FALSE] -> w229
        tunnel: w208 -> [w232 _]
        frame False {
          # "Only start if no errors"
        }
        frame True {
          # "Always start program"
        }
      }
      n61 = call "DAISY_Polarity_sign_array.vi"("error in (no error)"=w200, "BoardHandles"=w201) -> ("Errors Out"=w197:errorcluster[], "Polarity signs"=w199:i32[], "Board Handles Out"=w198:T7)  [unwired: 7 in]
    }
  }
  n62 = To Double Precision Float(number=w25) -> (double precision float=w10:dbl)
  n63 = Build Array(w25) -> (w34:timestamp[])
  n64 = Build Array(w10, w10) -> (w24:dbl[])
  n65 = case shown="False" w27 {
    selector: w27 -> [_ w1106]
    tunnel: [_ w1106] -> _
    tunnel: w38 -> [w251 _]
    tunnel: w37 -> [w256 _]
    tunnel: w15 -> [w255 _]
    tunnel: w36 -> [w252 w1104]
    tunnel: w34 -> [w254 _]
    tunnel: [w253 timestamp[] []] -> w30
    tunnel: w26 -> [w247 _]
    tunnel: w24 -> [w250 _]
    tunnel: [w249 w1104] -> w23
    tunnel: w22 -> [w248 _]
    tunnel: w20 -> [w246 w1103]
    tunnel: [w245 w1100] -> w19
    tunnel: [w244 w1103] -> w18
    tunnel: w12 -> [w243 w1102]
    tunnel: [w242 w1102] -> w11
    tunnel: w10 -> [w241 _]
    tunnel: w10 -> [w240 _]
    tunnel: w7 -> [w239 w1101]
    tunnel: [w238 w1101] -> w6
    tunnel: w5 -> [w237 _]
    tunnel: w3 -> [w236 w1100]
    tunnel: w2 -> [w235 w1099]
    tunnel: [w234 w1099] -> w1
    frame False {
      # "NI 9226"
      # "NI 9216"
      # "NI 9207"
      # "CAEN 1 & 2"
      # "Lakeshore"
      n66 = while {
        shift-right: [w272] -> _
        shift-left: w256 -> [w308]
        shift-right: [w285] -> _
        shift-left: w255 -> [w299]
        shift-right: [w277] -> w253
        shift-left: w254 -> [w305]
        shift-right: [w300] -> w245
        shift-left: w236 -> [w294]
        shift-right: [w302] -> _
        shift-left: w251 -> [w304]
        shift-right: [w301] -> w249
        shift-left: w252 -> [w303]
        shift-right: [w281] -> _
        shift-left: w247 -> [w296]
        shift-right: [w283] -> _
        shift-left: w247 -> [w297]
        shift-right: [w279] -> _
        shift-left: w250 -> [w295]
        shift-right: [w267] -> _
        shift-left: w248 -> [w293]
        shift-right: [w291] -> w244
        shift-left: w246 -> [w292]
        shift-right: [w289] -> w242
        shift-left: w243 -> [w290]
        shift-right: [w265] -> _
        shift-left: w241 -> [w266]
        shift-right: [w262] -> _
        shift-left: w240 -> [w263]
        shift-right: [w260] -> w238
        shift-left: w239 -> [w261]
        tunnel: w237 -> [w259]
        shift-right: [w257] -> w234
        shift-left: w235 -> [w258]
        stop <- w306 stop-if-true
        # "9226 (T)"
        # "Email timer"
        # "Alarm timer"
        # "Alarm status"
        # "LakeShore"
        # "9216 x2 (T)"
        # "9207 (V, mA)"
        # "HV supply altered?"
        # "Setpoint"
        # "Anode timing"
        # "Anode timers"
        # "Integrated flow"
        # "Flow"
        # "Flow"
        # "Integrated Flow"
        # "TOBA"
        # "Array of times"
        # "Latest HV read-outs"
        # "Time per cycle (s)"
        # "Cycle number"
        # "HV values: VSet, Vmax, IMax"
        # "HV values"
        # "TOBA"
        n67 = stacked-sequence {
          seq-local: [_ _ w484 _ _ _ _ _ _ _] -> [_ _ _ w596 _ _ _ _ _ _]
          seq-local: ["Time per cycle (s)" _ _ _ _ _ _ _ _ _] -> [_ _ _ _ _ _ w805 _ _ _]
          seq-local: [_ _ w468 _ _ _ _ _ _ _] -> [_ _ _ _ _ _ w803 _ _ _]
          seq-local: [_ w409 _ _ _ _ _ _ _ _] -> [_ _ _ _ w669 w788 _ _ _ _]
          seq-local: [_ _ w480 _ _ _ _ _ _ _] -> [_ _ _ w592 _ _ _ _ _ _]
          seq-local: [_ w402 _ _ _ _ _ _ _ _] -> [_ _ _ _ _ _ w802 _ _ _]
          seq-local: [_ w397 _ _ _ _ _ _ _ _] -> [_ _ _ _ w691 w780 w800 w912 w942 w1028]
          seq-local: [_ w371 _ _ _ _ _ _ _ _] -> [_ _ _ _ w694 w783 w807 _ _ _]
          seq-local: [_ w385 _ _ _ _ _ _ _ _] -> [_ _ _ _ w693 w782 w801 _ _ _]
          seq-local: [_ _ _ _ _ _ _ w872 _ _] -> [_ _ _ _ _ _ _ _ w944 w1029]
          seq-local: [_ w372 _ _ _ _ _ _ _ _] -> [_ _ _ _ w680 _ w799 w870 w938 w1011]
          tunnel: [w333 _ _ _ _ _ _ _ _ _] -> w271
          tunnel: "stop" -> [w332 _ _ _ _ _ _ _ _ _]
          tunnel: w308 -> [w322 w398 _ _ _ _ _ _ _ _]
          tunnel: w299 -> [_ w399 _ _ w723 _ _ _ _ _]
          tunnel: [_ _ _ _ w678 _ _ _ _ _] -> w286
          tunnel: w305 -> [_ w378 _ _ _ _ _ _ _ _]
          tunnel: w294 -> [_ _ w474 w597 _ _ _ _ _ _]
          tunnel: w304 -> [_ _ _ _ _ _ _ _ _ _]
          tunnel: w303 -> [_ w411 _ _ _ _ _ w926 _ _]
          tunnel: [_ w412 _ _ _ _ _ _ _ _] -> w301
          tunnel: [_ _ w468 _ _ _ _ _ _ _] -> w302
          tunnel: [_ _ w461 _ _ _ _ _ _ _] -> w300
          tunnel: [_ _ _ _ w669 _ _ _ _ _] -> w278
          tunnel: w296 -> [_ _ _ _ _ w786 _ _ _ _]
          tunnel: w297 -> [_ _ _ _ _ w787 _ _ _ _]
          tunnel: w295 -> [_ _ _ w598 _ _ _ _ _ _]
          tunnel: [_ _ _ w593 _ _ _ _ _ _] -> w280
          tunnel: w293 -> [_ w405 _ _ _ _ _ _ _ _]
          tunnel: w292 -> [_ w404 _ _ _ _ _ w925 _ _]
          tunnel: [_ w400 _ _ _ _ _ _ _ _] -> w291
          tunnel: [_ _ _ _ _ w785 _ _ _ _] -> w282
          tunnel: [_ _ _ _ _ w784 _ _ _ _] -> w284
          tunnel: w290 -> [_ w384 _ _ _ _ _ w913 _ _]
          tunnel: [_ w380 _ _ _ _ _ _ _ _] -> w289
          tunnel: [_ _ _ _ _ _ _ _ w946 _] -> w267
          tunnel: w266 -> [_ _ _ _ _ _ _ _ w941 _]
          tunnel: [_ _ _ _ _ _ _ _ w939 _] -> w265
          tunnel: w263 -> [_ _ _ _ _ _ _ _ _ w1016]
          tunnel: [_ _ _ _ _ _ _ _ _ w1015] -> w262
          tunnel: w261 -> [_ w377 _ _ _ _ _ _ _ _]
          tunnel: [_ w373 _ _ _ _ _ _ _ _] -> w260
          tunnel: w259 -> [_ _ w471 _ _ _ _ _ _ _]
          tunnel: w258 -> [_ _ w473 w590 _ _ _ w869 _ _]
          tunnel: [_ _ w457 _ _ _ _ _ _ _] -> w257
          frame #0 {
            # "CAEN channel names\nupdater, real-time"
            # "Also, dumping ground for variables and controls that may be updated during run-time"
            # "CAEN needle gauges\nMin. and Max. ranges"
            # "To view documentation of modules, look for icons that have a \"Descr.\" label near them,\nright-click these and select \"Description and tip\". For example on frame 2, \"High Voltage\",\na \"Quotient and Remainder\" icon on the left-hand side may be checked out, to view the\ndocumentation for the \"Reading Voltages and Currents\" module, which uses that icon. \n\nIf all else fails, consult the user manual, National Instruments knowledge base or Google."
            # "Time to wait, in between cycles"
            # "If the program is stopped, a final cycle executes without delay."
            # "Waiting for \"interval time\" to have passed, to start new cycle"
            n68 = call "Is Value Changed.vim"("value"="Channel Names (CAEN)") -> ("changed or first call?"=w325:bool)
            n69 = case shown="True" w325 {
              tunnel: "Channel Names (CAEN)" -> [_ w339]
              frame False {
              }
              frame True {
                n70 = Index Array(array=w339) -> (element #1=→"CAEN 1.0":string, element #2=→"CAEN 1.1":string, element #3=→"CAEN 1.2":string, element #4=→"CAEN 1.3":string, element #5=→"CAEN 2.0":string, element #6=→"CAEN 2.1":string, element #7=→"CAEN 2.2 2":string, element #8=→"CAEN 2.3 2":string)  [unwired: 8 in]
                "CAEN Ch. Names" <- w339
                "Channel Names" <- w339
                "Channel Names" <- w339
              }
            }
            n71 = Increment(x=w322) -> (x+1=w333:i32)
            n72 = local read "Channel Names (9207, ai0:7)"() -> (w323:string[])
            n73 = To Long Integer(number="Detector pressure input:") -> (32bit integer=→"Det.P input #":i32)
            n74 = To Long Integer(number="Flow meter input:") -> (32bit integer=→"Flow input #":i32)
            n75 = call "Is Value Changed.vim"("value"=w323) -> ("changed or first call?"=w324:bool)
            n76 = case shown="True" w324 {
              tunnel: w323 -> [_ w335]
              frame False {
                # ":D"
              }
              frame True {
                n77 = for {
                  tunnel: w335 -> [w338] mode=indexing
                  tunnel: [w336] -> w334 mode=indexing
                  i -> [w337]
                  n78 = Bundle("Or give name if \"Other\""=w338, w337) -> (w336:cluster{"Or give name if \"Other\"":string, i32})  [unwired: 1 in]
                }
                n79 = property on="Detector pressure input:" class="Ring (strict)"("StringsAndValues[]"=w334) -> ()  [unwired: 2 in, 2 out]
                n80 = property on="Flow meter input:" class="Ring (strict)"("StringsAndValues[]"=w334) -> ()  [unwired: 2 in, 2 out]
              }
            }
            n81 = case shown="False" w332 {
              tunnel: "Time per cycle (s)" -> [w364 _]
              frame False {
                n82 = while {
                  tunnel: w364 -> [w366]
                  stop <- w368 stop-if-true
                  n83 = call "Elapsed Time"("Time Target (s)"=w366) -> ("Elapsed Time (s)"=w367:dbl, "Time has Elapsed"=w368:bool)  [unwired: 11 in, 6 out]
                  n84 = Subtract(x=w366, y=w367) -> (x-y=→"Time until next cycle":dbl)
                }
              }
              frame True {
              }
            }
            n85 = stacked-sequence {
              frame #0 {
                n86 = property on="CAEN 1.0" class="Knob (strict)"("Scale.Minimum"="Scale.Range:Minimum", "Scale.Maximum"="Scale.Range:Maximum") -> ()  [unwired: 2 in, 2 out]
                n87 = property on="CAEN 1.1" class="Knob (strict)"("Scale.Minimum"="Scale.Range:Minimum 2", "Scale.Maximum"="Scale.Range:Maximum 2") -> ()  [unwired: 2 in, 2 out]
              }
              frame #1 {
                n88 = property on="CAEN 1.2" class="Knob (strict)"("Scale.Minimum"="Scale.Range:Minimum 3", "Scale.Maximum"="Scale.Range:Maximum 3") -> ()  [unwired: 2 in, 2 out]
                n89 = property on="CAEN 1.3" class="Knob (strict)"("Scale.Maximum"="Scale.Range:Maximum 4", "Scale.Minimum"="Scale.Range:Minimum 4") -> ()  [unwired: 2 in, 2 out]
              }
              frame #2 {
                n90 = property on="CAEN 2.1" class="Knob (strict)"("Scale.Maximum"="Scale.Range:Maximum 6", "Scale.Minimum"="Scale.Range:Minimum 6") -> ()  [unwired: 2 in, 2 out]
                n91 = property on="CAEN 2.0" class="Knob (strict)"("Scale.Maximum"="Scale.Range:Maximum 5", "Scale.Minimum"="Scale.Range:Minimum 5") -> ()  [unwired: 2 in, 2 out]
              }
              frame #3 {
                n92 = property on="CAEN 2.2" class="Knob (strict)"("Scale.Maximum"="Scale.Range:Maximum 7", "Scale.Minimum"="Scale.Range:Minimum 7") -> ()  [unwired: 2 in, 2 out]
                n93 = property on="CAEN 2.3" class="Knob (strict)"("Scale.Maximum"="Scale.Range:Maximum 8", "Scale.Minimum"="Scale.Range:Minimum 8") -> ()  [unwired: 2 in, 2 out]
              }
            }
            "Cycle number" <- w322
          }
          frame #1 {
            # "Module 3 tasks + status"
            # "Module 0, 1 tasks + status"
            # "Lake Shore task + status"
            # "DAQmx Read above will replace dummy data below,\nonce the 9216 modules are functioning"
            # "Descr"
            # "NI 9207 8x V, 8x mA"
            # "Case to ignore runtime errors; unpack later"
            # "Module 2 tasks+status"
            # "Temps (NI)"
            # "9216 T     (NI) x16\n9207 V     (NI)  x8\n9207 mA (NI)  x8\nTemp        (LS)  x2\nHeater %           x1"
            # "Temp A, Temp B, heater power"
            # "Measurements and conversions"
            n94 = case shown="True" "Run lakeshore?" {
              tunnel: [w435 w446] -> w412
              tunnel: w411 -> [w435 w445]
              tunnel: [-273.0 ("Input A") w444] -> w408
              tunnel: [-273.0 ("Input B") w443] -> w407
              tunnel: [73.0 ("Heater 1 (%)") w442] -> w406
              tunnel: w405 -> [_ w440]
              tunnel: [-274.0 "Setpoint (°C)"] -> w402
              frame False {
                # "Dummy data"
              }
              frame True {
                # "LS output"
                # "P\nI\nD"
                n95 = Select(t=0, s=w440, f="Heater range") -> (s? t:f=w437:i32)
                "heater" <- w437
                n96 = Unbundle("PID settings") -> ("P"=w451:dbl, "I"=w450:dbl, "D"=w449:dbl)
                n97 = Unbundle(w445) -> ("VISA resource name out"=w453:refnum<visa-resource-name>, "error out"=w452:errorcluster)
                n98 = call "Lakeshore subVI.vi"("Setpoint"="Setpoint (°C)", "Rate (D) (X.X %)"=w449, "Range"=w437, "Reset (I) (XX.X)"=w450, "Gain (P) (XX.X)"=w451, "error in (no error)"=w452, "VISA resource name"=w453) -> ("Input B"=w443:dbl, "Input A"=w444:dbl, "error out"=w447:errorcluster, "VISA resource name out"=w448:refnum<visa-resource-name>, "Heater 1 (%)"=w442:dbl)
                "Lakeshore" <- w447
                n99 = Bundle("VISA resource name out"=w448, "error out"=w447) -> (w446:T6)  [unwired: 1 in]
              }
            }
            n100 = Get Date/Time In Seconds() -> (seconds since 1Jan1904=w410:timestamp)
            n101 = Quotient & Remainder(x=w398, y="Read T every N cycles") -> (x-y*floor(x/y)=w401:i32)  [unwired: 1 out]
            n102 = Unbundle(w384) -> ("task out"=w383:refnum<k21>, "error out"=w382:errorcluster)
            n103 = Build Array (concatenate)(w378, w410) -> (w409:timestamp[])
            n104 = Unbundle(w404) -> ("task out"=w389:refnum<k21>, "error out"=w388:errorcluster)
            n105 = case shown="0" w401 {
              tunnel: w399 -> [_ w428]
              tunnel: [w421 w424] -> w371
              tunnel: w398 -> [w420 _]
              frame 0 {
                # "Dummy data"
                # "New temperatures"
                n106 = Add(x=w420, y=-95.0 ("element")) -> (x+y=w423:dbl)
                n107 = Initialize Array(w423, 16) -> (w421:dbl[])
              }
              frame 1, Default {
                # "Gets 1st 16 Col's\nfrom last row:\nPrevious 16 temps."
                # "Get previous temps"
                n108 = Array Size(array=w428) -> (size(s)=w430:i32[])
                n109 = Index Array(array=w430, index=0) -> (element=w431:i32)
                n110 = Decrement(x=w431) -> (x-1=w427:i32)
                n111 = Index Array(array=w428, index (row)=w427) -> (element=w426:dbl[])  [unwired: 1 in]
                n112 = Array Subset(array=w426, length=16) -> (w424:dbl[])  [unwired: 1 in]
              }
            }
            n113 = call-poly <vilib>:"DAQmx Read.vi"("task/channels in"=w383, "error in"=w382) -> ("task out"=w370:refnum<k21>, "data"=→"PT100 data":dbl[], "error out"=w381:errorcluster)  [unwired: 11 in]
            "NI 9216 x2" <- w381
            n114 = call-poly <vilib>:"DAQmx Read.vi"("task/channels in"=w389, "error in"=w388) -> ("task out"=w387:refnum<k21>, "data"=w396:dbl[], "error out"=w386:errorcluster)  [unwired: 11 in]
            "Raw readouts (V, mA)" <- w396
            "NI 9207" <- w386
            n115 = Build Array (concatenate)("Offsets\nsubtracted", "Offsets\nsubtracted") -> (w390:dbl[])
            n116 = Build Array (concatenate)("Multipliers", "Multipliers") -> (w393:dbl[])
            n117 = for {
              tunnel: w390 -> [w418] mode=indexing
              tunnel: w396 -> [w417] mode=indexing
              tunnel: w393 -> [w415] mode=indexing
              tunnel: [w414] -> w397 mode=indexing
              n118 = Subtract(x=w417, y=w418) -> (x-y=w416:dbl)
              n119 = Multiply(x=w416, y=w415) -> (x*y=w414:dbl)
            }
            n120 = Bundle("task out"=w370, "error out"=w381) -> (w380:T5)  [unwired: 1 in]
            n121 = Bundle("task out"=w387, "error out"=w386) -> (w400:T5)  [unwired: 1 in]
            n122 = Build Array(w408, w407, w406) -> (w385:dbl[])
            "LakeShore readings" <- w385
            n123 = Unbundle(w377) -> ("task out"=w369:refnum<k21>, "error out"=w376:errorcluster)
            n124 = call-poly <vilib>:"DAQmx Read.vi"("task/channels in"=w369, "error in"=w376) -> ("task out"=w375:refnum<k21>, "data"=w372:dbl[], "error out"=w374:errorcluster)  [unwired: 11 in]
            "NI 9226" <- w374
            "PT1000 data" <- w372
            n125 = Bundle("task out"=w375, "error out"=w374) -> (w373:T5)  [unwired: 1 in]
          }
          frame #2 {
            # "Alter voltages if button clicked"
            # "Descr."
            # "VMON1  x4 \nVMON2  x4\nIMON1    x4\nIMON2    x4"
            # "Needle gauge Voltage displays"
            # "High Voltage"
            n126 = for {
              tunnel: w474 -> [w589] mode=indexing
              tunnel: w473 -> [w588] mode=indexing
              tunnel: [w587] -> w466 mode=indexing
              tunnel: [w586] -> w465 mode=indexing
              tunnel: [w585] -> w472 mode=concatenating
              tunnel: [w584] -> w469 mode=concatenating
              n127 = call "Read_supply_with_boardhandle.vi"("error in (no error)"=w588, "BoardHandle"=w589) -> ("error out"=w586:errorcluster, "IMon values (uA)"=w584:dbl[], "VMon values (V)"=w585:dbl[], "BoardHandle out"=w587:T8)  [unwired: 6 in]
            }
            "IMon (uA)" <- w469
            n128 = Build Array (concatenate)("VSet (V)", "VMax (V)", "IMax (uA)") -> (w484:dbl[])
            n129 = case shown="True" "Query HV status" {
              tunnel: w466 -> [w567 w575]
              tunnel: w465 -> [w566 w574]
              tunnel: [w567 w569] -> w463
              tunnel: [w566 w568] -> w462
              frame False {
              }
              frame True {
                n130 = for {
                  tunnel: w575 -> [w580] mode=indexing
                  tunnel: w574 -> [w579] mode=indexing
                  tunnel: [w578] -> w569 mode=indexing
                  tunnel: [w577] -> w568 mode=indexing
                  tunnel: [w576] -> w573 mode=concatenating
                  n131 = call <instrlib>:"Channel Status.vi"("error in (no error)"=w579, "BoardHandle"=w580) -> ("error out"=w577:errorcluster, "Channel Status Array"=w576:T2, "BoardHandle out"=w578:T4)  [unwired: 7 in]
                }
                n132 = Delete From Array(array=w573, length=4) -> (deleted portion=→"CAEN 1":T2, array with subset deleted=→"CAEN 2":T2)  [unwired: 1 in]
              }
            }
            n133 = Or(x="Kill all channels", y="Kill voltage") -> (x .or. y?=w475:bool)
            n134 = for {
              tunnel: w472 -> [w582] mode=indexing
              tunnel: w471 -> [w583] mode=indexing
              tunnel: [w581] -> w470 mode=indexing
              n135 = Multiply(x=w583, y=w582) -> (x*y=w581:dbl)
            }
            "Voltages" <- w470
            "Vmon (V)" <- w470
            n136 = Build Array("Apply Voltage", "Set to zero (ramp down)", w475) -> (w480:bool[])
            n137 = Build Array (concatenate)(w470, w469) -> (w468:dbl[])
            n138 = Search 1D Array(1D array=w480, element=TRUE) -> (index of element=w464:i32)  [unwired: 1 in]
            n139 = case shown="2" w464 {
              tunnel: w463 -> [w497 w526 w551 w565]
              tunnel: w462 -> [w496 w525 w550 w564]
              tunnel: [w492 w522 w549 w565] -> w461
              tunnel: [w491 w521 w548 w564] -> w457
              tunnel: "VSet (V)" -> [w495 _ _ _]
              tunnel: "VMax (V)" -> [w494 w524 _ _]
              tunnel: "IMax (uA)" -> [w493 w523 _ _]
              frame 0 {
                # "Apply settings"
                n140 = for {
                  N: 2 -> [_]
                  tunnel: w497 -> [w511] mode=indexing
                  tunnel: w496 -> [w510] mode=indexing
                  tunnel: w495 -> [w507]
                  tunnel: w494 -> [w505]
                  tunnel: w493 -> [w503]
                  tunnel: [w500] -> w492 mode=indexing
                  tunnel: [w499] -> w491 mode=indexing
                  i -> [w509]
                  n141 = Multiply(x=4, y=w509) -> (x*y=w504:i32)
                  n142 = Array Subset(array=w505, index=w504) -> (w502:dbl[])  [unwired: 1 in]
                  n143 = Array Subset(array=w507, index=w504) -> (w506:dbl[])  [unwired: 1 in]
                  n144 = Array Subset(array=w503, index=w504) -> (w501:dbl[])  [unwired: 1 in]
                  n145 = for {
                    N: 4 -> [_]
                    tunnel: w511 -> [w519]
                    tunnel: w510 -> [w518]
                    tunnel: w506 -> [w517] mode=indexing
                    tunnel: w502 -> [w516] mode=indexing
                    tunnel: w501 -> [w515] mode=indexing
                    tunnel: [w514] -> w500
                    tunnel: [w513] -> w499
                    i -> [w520]
                    n146 = call "Set_supply_with_boardhandle.vi"("Current Limit (0.00 uA)"=w515, "Channel (0)"=w520, "error in (no error)"=w518, "Voltage Max (0.0 V)"=w516, "Voltage Level (0.0 V)"=w517, "BoardHandle"=w519) -> ("error out"=w513:errorcluster, "BoardHandle out"=w514:T8)  [unwired: 4 in]
                  }
                }
              }
              frame 1 {
                # "Set to zero"
                n147 = for {
                  N: 2 -> [_]
                  tunnel: w526 -> [w538] mode=indexing
                  tunnel: w525 -> [w537] mode=indexing
                  tunnel: w524 -> [w534]
                  tunnel: w523 -> [w532]
                  tunnel: [w529] -> w522 mode=indexing
                  tunnel: [w528] -> w521 mode=indexing
                  i -> [w536]
                  n148 = Multiply(x=4, y=w536) -> (x*y=w533:i32)
                  n149 = Array Subset(array=w534, index=w533) -> (w531:dbl[])  [unwired: 1 in]
                  n150 = Array Subset(array=w532, index=w533) -> (w530:dbl[])  [unwired: 1 in]
                  n151 = for {
                    N: 4 -> [_]
                    tunnel: w538 -> [w546]
                    tunnel: w537 -> [w545]
                    tunnel: w531 -> [w544] mode=indexing
                    tunnel: w530 -> [w543] mode=indexing
                    tunnel: [w542] -> w529
                    tunnel: [w541] -> w528
                    i -> [w547]
                    n152 = call "Set_supply_with_boardhandle.vi"("Current Limit (0.00 uA)"=w543, "Channel (0)"=w547, "error in (no error)"=w545, "Voltage Max (0.0 V)"=w544, "Voltage Level (0.0 V)"=0, "BoardHandle"=w546) -> ("error out"=w541:errorcluster, "BoardHandle out"=w542:T8)  [unwired: 4 in]
                  }
                }
              }
              frame 2 {
                # "Kill all channels"
                n153 = for {
                  N: 2 -> [_]
                  tunnel: w551 -> [w556] mode=indexing
                  tunnel: w550 -> [w555] mode=indexing
                  tunnel: [w554] -> w549 mode=indexing
                  tunnel: [w553] -> w548 mode=indexing
                  n154 = for {
                    N: 4 -> [_]
                    tunnel: w556 -> [w562]
                    tunnel: w555 -> [w561]
                    tunnel: [w560] -> w554
                    tunnel: [w559] -> w553
                    i -> [w563]
                    w558 = 0
                    n155 = call "Set_supply_with_boardhandle.vi"("Current Limit (0.00 uA)"=w558, "Channel (0)"=w563, "error in (no error)"=w561, "Voltage Max (0.0 V)"=w558, "Voltage Level (0.0 V)"=w558, "BoardHandle"=w562) -> ("error out"=w559:errorcluster, "BoardHandle out"=w560:T8)  [unwired: 4 in]
                  }
                }
              }
              frame 3, Default {
                # "Do nothing"
              }
            }
            n156 = Index Array(array=w468) -> (element #1=→"CAEN 1.0":dbl, element #2=→"CAEN 1.1":dbl, element #3=→"CAEN 1.2":dbl, element #4=→"CAEN 1.3":dbl, element #5=→"CAEN 2.0":dbl, element #6=→"CAEN 2.1":dbl, element #7=→"CAEN 2.2":dbl, element #8=→"CAEN 2.3":dbl)  [unwired: 8 in]
            n157 = Index Array(array=w457) -> (element #1=→"CAEN 1":errorcluster, element #2=→"CAEN 2":errorcluster)  [unwired: 2 in]
          }
          frame #3 {
            # "Descr."
            # "Reset anode"
            n158 = Or Array Elements(Boolean array=w592) -> (logical OR=w591:bool)
            n159 = case shown="True" "Reset anode\nperiodically?" {
              tunnel: w598 -> [_ w607]
              tunnel: w597 -> [_ w614]
              tunnel: w596 -> [_ w619]
              tunnel: w591 -> [_ w605]
              tunnel: [w599 w606] -> w593
              tunnel: w590 -> [_ w603]
              frame False {
                # "Anode Reset Routine inactive:\nkeep timers up to date so activating\nroutine will correctly initiate the timers."
                n160 = Get Date/Time In Seconds() -> (seconds since 1Jan1904=w601:timestamp)
                n161 = To Double Precision Float(number=w601) -> (double precision float=w600:dbl)
                n162 = Build Array(w600, w600) -> (w599:dbl[])
              }
              frame True {
                n163 = case shown="\"CAEN 2\"" "CAEN unit selector" {
                  tunnel: w614 -> [w634 w640]
                  tunnel: [0 4] -> w612
                  tunnel: [w632 w638] -> w604
                  tunnel: w603 -> [w631 w636]
                  tunnel: [w630 w635] -> w602
                  frame "CAEN 1", Default {
                    n164 = Index Array(array=w634) -> (element=w632:T4)  [unwired: 1 in]
                    n165 = Index Array(array=w631) -> (element=w630:errorcluster)  [unwired: 1 in]
                  }
                  frame "CAEN 2" {
                    n166 = Index Array(array=w640, index=1) -> (element=w638:T4)
                    n167 = Index Array(array=w636, index=1) -> (element=w635:errorcluster)
                  }
                }
                n168 = call "anode_timing.vi"("Keep off for X seconds"="Keep off for X seconds", "Array of timers"=w607, "Kill every Y minutes"="Kill every Y minutes") -> ("Time to kill"=w621:bool, "Time until reset"=→"Seconds until \nanode reset":dbl, "Time until autokill"=→"Seconds until \nanode autokill":dbl, "Time to reset"=w622:bool)  [unwired: 5 in]
                "Killed" <- w621
                "Restarted" <- w622
                n169 = Add(x=w612, y="Anode ch.") -> (x+y=w610:i32)
                n170 = Build Array(w621, w622, w605) -> (w625:bool[])
                n171 = Add(x=w610, y=8) -> (x+y=w615:i32)
                n172 = Add(x=w610, y=16) -> (x+y=w616:i32)
                n173 = Search 1D Array(1D array=w625, element=TRUE) -> (index of element=w624:i32)  [unwired: 1 in]
                n174 = Index Array(array=w619, index #1=w610, index #2=w615, index #3=w616) -> (element #1=w628:dbl, element #2=w626:dbl, element #3=w627:dbl)
                n175 = case shown="0" w624 {
                  tunnel: w628 -> [_ w656 _ _]
                  tunnel: w626 -> [w648 w657 _ _]
                  tunnel: w627 -> [w647 w658 _ _]
                  tunnel: "Anode ch." -> [w644 w659 _ _]
                  tunnel: w607 -> [w650 _ _ w668]
                  tunnel: [w649 w662 w665 w668] -> w606
                  tunnel: w604 -> [w645 w660 _ _]
                  tunnel: w602 -> [w646 w661 _ _]
                  frame 0 {
                    # "Set Anode Voltage to zero,\nreset the 1st timer"
                    # "Anode Vset to zero"
                    n176 = Get Date/Time In Seconds() -> (seconds since 1Jan1904=w653:timestamp)
                    n177 = call "Set_supply_with_boardhandle.vi"("Current Limit (0.00 uA)"=w647, "Channel (0)"=w644, "error in (no error)"=w646, "Voltage Max (0.0 V)"=w648, "Voltage Level (0.0 V)"=0, "BoardHandle"=w645) -> ("error out"=w643:errorcluster)  [unwired: 4 in, 1 out]
                    n178 = Index Array(array=w650, index=1) -> (element=w651:dbl)
                    n179 = To Double Precision Float(number=w653) -> (double precision float=w652:dbl)
                    n180 = Build Array(w652, w651) -> (w649:dbl[])
                    n181 = call <vilib>:"Simple Error Handler.vi"("error in (no error)"=w643) -> ()  [unwired: 4 in, 5 out]
                  }
                  frame 1 {
                    # "Set Anode Voltage to defined value,\nreset both timers"
                    # "Anode Vset applied"
                    n182 = Get Date/Time In Seconds() -> (seconds since 1Jan1904=w664:timestamp)
                    n183 = call "Set_supply_with_boardhandle.vi"("Current Limit (0.00 uA)"=w658, "Channel (0)"=w659, "error in (no error)"=w661, "Voltage Max (0.0 V)"=w657, "Voltage Level (0.0 V)"=w656, "BoardHandle"=w660) -> ("error out"=w655:errorcluster)  [unwired: 4 in, 1 out]
                    n184 = To Double Precision Float(number=w664) -> (double precision float=w663:dbl)
                    n185 = Build Array(w663, w663) -> (w662:dbl[])
                    n186 = call <vilib>:"Simple Error Handler.vi"("error in (no error)"=w655) -> ()  [unwired: 4 in, 5 out]
                  }
                  frame 2 {
                    # "Change Voltage button pressed"
                    # "Reset both timers"
                    n187 = Get Date/Time In Seconds() -> (seconds since 1Jan1904=w667:timestamp)
                    n188 = To Double Precision Float(number=w667) -> (double precision float=w666:dbl)
                    n189 = Build Array(w666, w666) -> (w665:dbl[])
                  }
                  frame 3, Default {
                    # "Timers stay at previous value,\nso difference between those and\ncurrent time keeps incrementing"
                    # "No event"
                  }
                }
              }
            }
            n190 = To Time Stamp(1:w593) -> (0:→"Anode timers":timestamp[])
            "?" <- "Reset anode\nperiodically?"
          }
          frame #4 {
            # "Det. P"
            # "Flow"
            # "Flexibly acquire indices"
            # "Plots 9207 output vs time"
            # "Descr."
            # "Moving averages"
            # "Historic graphs: Phase, 9207 ai, Flow, Heater, Temperature"
            # "Non-historic Temperature + Det. Pressure"
            # "Updated TOBA >>>"
            # "Descr."
            # "Latest Detector Pressure"
            # "Plots individual lists of Temp. vs. t"
            # "Plots and moving averages"
            n191 = Build Array (concatenate)(w694, w680, w691, w693) -> (w722:dbl[])
            n192 = Build Array (concatenate)(w723, w722) -> (w678:dbl[][])
            "TOBA appended" <- w678
            n193 = Array Size(array=w691) -> (size(s)=w690:i32)
            n194 = Array Size(array=w680) -> (size(s)=w692:i32)
            n195 = Array Size(array=w694) -> (size(s)=w681:i32)
            n196 = Add(x=w681, y=w692) -> (x+y=w676:i32)
            n197 = Add(x=w676, y=w690) -> (x+y=w689:i32)
            n198 = local read "Flow input #"() -> (w700:i32)
            n199 = local read "Det.P input #"() -> (w701:i32)
            n200 = Add(x=w689, y=2 ("disabled index (col)")) -> (x+y=w687:i32)
            n201 = Equal?(x=666, y="Temperature channel selector") -> (x = y?=w716:bool)
            n202 = Index Array(array=w678, index (col)=w687) -> (element=w686:dbl[])  [unwired: 1 in]
            n203 = case shown="True" w716 {
              tunnel: w680 -> [w761 w762]
              tunnel: [w760 w763] -> w714
              tunnel: "Temperature channel selector" -> [w759 _]
              frame False {
                n204 = Index Array(array=w761, index=w759) -> (element=w760:dbl)
              }
              frame True {
                n205 = Add Array Elements(numeric array=w762) -> (sum=w764:dbl)
                n206 = Array Size(array=w762) -> (size(s)=w765:i32)
                n207 = Divide(x=w764, y=w765) -> (x/y=w763:dbl)
              }
            }
            n208 = Add(x=w701, y=w676) -> (x+y=w710:i32)
            n209 = Add(x=w676, y=w700) -> (x+y=w708:i32)
            n210 = Bundle(w669, w686) -> (w683:cluster{timestamp[], dbl[]})  [unwired: 1 in]
            n211 = Build Array(w683) -> (→"Heater power (%)":cluster{timestamp[], dbl[]}[])
            n212 = Add(x=w681, y="Temperature Channel Selector") -> (x+y=w684:i32)
            n213 = Index Array(array=w678, index (col) #1=w710, index (col) #2=w708) -> (element #1=w709:dbl[], element #2=w698:dbl[])  [unwired: 2 in]
            n214 = local read "Det.P input #"() -> (w702:i32)
            n215 = Index Array(array=w678, index (col)=w684) -> (element=w713:dbl[])  [unwired: 1 in]
            n216 = for {
              N: 8 -> [_]
              tunnel: w678 -> [w752]
              tunnel: w669 -> [w745]
              tunnel: [w749] -> w706 mode=indexing
              tunnel: [w744] -> w705 mode=indexing
              tunnel: w676 -> [w742]
              i -> [w748]
              n217 = Add(x=w742, y=8) -> (x+y=w741:i32)
              n218 = Add(x=w742, y=w748) -> (x+y=w751:i32)
              n219 = Add(x=w748, y=w741) -> (x+y=w747:i32)
              n220 = Index Array(array=w752, index (col) #1=w751, index (col) #2=w747) -> (element #1=w750:dbl[], element #2=w746:dbl[])  [unwired: 2 in]
              n221 = Bundle(w745, w750) -> (w749:cluster{timestamp[], dbl[]})  [unwired: 1 in]
              n222 = Bundle(w745, w746) -> (w744:cluster{timestamp[], dbl[]})  [unwired: 1 in]
            }
            "9207 (ai 0:7, Volts)" <- w706
            "9207 (ai 8:15, Amperes)" <- w705
            n223 = Bundle(w713, w709) -> (w727:cluster{dbl[], dbl[]})  [unwired: 1 in]
            n224 = Index Array(array=w691, index=w702) -> (element=w728:dbl)
            n225 = call "moving_avg.vi"("N samples"="N samples", "Array"=w709) -> ("Numeric"=→"Detector Pressure":dbl)  [unwired: 9 in]
            n226 = call "moving_avg.vi"("N samples"="N samples", "Array"=w698) -> ("Numeric"=→"Average Flow (SLPM)":dbl)  [unwired: 9 in]
            n227 = Bundle(w669, w698) -> (w725:cluster{timestamp[], dbl[]})  [unwired: 1 in]
            n228 = Build Array(w727) -> (→"Historical Large Phase Diagram":cluster{dbl[], dbl[]}[])
            n229 = Bundle("Waveform"=w714, w728) -> (w732:cluster{"Waveform":dbl, dbl})  [unwired: 1 in]
            n230 = Build Array(w725) -> (→"Flow (SLPM)":cluster{timestamp[], dbl[]}[])
            n231 = Build Array(w732) -> (→"Phase Diagram":cluster{"Waveform":dbl, dbl}[])
            n232 = for {
              N: w681 -> [_]
              tunnel: w669 -> [w777]
              tunnel: [w776] -> w733 mode=indexing
              tunnel: w678 -> [w775]
              i -> [w773]
              n233 = Index Array(array=w775, index (col)=w773) -> (element=w774:dbl[])  [unwired: 1 in]
              n234 = Bundle(w777, w774) -> (w776:cluster{timestamp[], dbl[]})  [unwired: 1 in]
            }
            "Setup Temperature (9216 0:15, °C)" <- w733
            n235 = Increment(x=w676) -> (x+1=w677:i32)
            n236 = Array Size(array=w680) -> (size(s)=w679:i32)
            n237 = Equal?(x=666, y="Temperature Channel Selector") -> (x = y?=w718:bool)
            n238 = Index Array(array=w678, index (col) #1=w676, index (col) #2=w677) -> (element #1=w675:dbl[], element #2=w674:dbl[])  [unwired: 2 in]
            n239 = local read "Channel Names (9207, ai0:7)"() -> (w703:string[])
            n240 = local read "Channel Names (9207, ai8:15)"() -> (w704:string[])
            n241 = case shown="False" w718 {
              tunnel: w680 -> [w768 w769]
              tunnel: [w767 w770] -> w721
              tunnel: "Temperature Channel Selector" -> [w766 _]
              frame False {
                n242 = Index Array(array=w768, index=w766) -> (element=w767:dbl)
              }
              frame True {
                n243 = Add Array Elements(numeric array=w769) -> (sum=w771:dbl)
                n244 = Array Size(array=w769) -> (size(s)=w772:i32)
                n245 = Divide(x=w771, y=w772) -> (x/y=w770:dbl)
              }
            }
            n246 = for {
              N: w679 -> [_]
              tunnel: w669 -> [w740]
              tunnel: [w739] -> w673 mode=indexing
              tunnel: w678 -> [w738]
              tunnel: w681 -> [w734]
              i -> [w735]
              n247 = Add(x=w734, y=w735) -> (x+y=w736:i32)
              n248 = Index Array(array=w738, index (col)=w736) -> (element=w737:dbl[])  [unwired: 1 in]
              n249 = Bundle(w740, w737) -> (w739:cluster{timestamp[], dbl[]})  [unwired: 1 in]
            }
            n250 = Bundle(w669, w675) -> (w672:cluster{timestamp[], dbl[]})  [unwired: 1 in]
            n251 = Bundle(w669, w674) -> (w671:cluster{timestamp[], dbl[]})  [unwired: 1 in]
            n252 = call "Is Value Changed.vim"("value"=w704) -> ("changed or first call?"=w711:bool)
            n253 = call "Is Value Changed.vim"("value"=w703) -> ("changed or first call?"=w712:bool)
            n254 = case shown="True" w711 {
              tunnel: w704 -> [_ w753]
              frame False {
              }
              frame True {
                n255 = for {
                  tunnel: w753 -> [w754] mode=indexing
                  i -> [w755]
                  n256 = property on="9207 (ai 8:15, Amperes)" class="XYGraph (strict)"("Active Plot"=w755, "Plot.Plot Name"=w754) -> ()  [unwired: 2 in, 2 out]
                }
              }
            }
            n257 = case shown="True" w712 {
              tunnel: w703 -> [_ w756]
              frame False {
              }
              frame True {
                n258 = for {
                  tunnel: w756 -> [w757] mode=indexing
                  i -> [w758]
                  n259 = property on="9207 (ai 0:7, Volts)" class="XYGraph (strict)"("Active Plot"=w758, "Plot.Plot Name"=w757) -> ()  [unwired: 2 in, 2 out]
                }
              }
            }
            n260 = Bundle("Waveform"=w721, w728) -> (w730:cluster{"Waveform":dbl, dbl})  [unwired: 1 in]
            n261 = Build Array (concatenate)(w673, w672, w671) -> (→"Low Temperature (9226 0:7 and LakeShore A;B, °C)":cluster{timestamp[], dbl[]}[])
            n262 = Build Array(w730) -> (→"Large Phase Diagram":cluster{"Waveform":dbl, dbl}[])
          }
          frame #5 {
            # "Temp A, Temp B, Heater%"
            # "Temperatures x16\nTo indicators on the physical schematic"
            # "Individual latest 9207 readings.\nIndicators go here. Array is 1x16,\nitems have been converted using\nthe offsets and multipliers"
            # "Displays"
            n263 = local read "Flow input #"() -> (w781:i32)
            n264 = case shown="False" "Reset?" {
              tunnel: [w793 0.0] -> w789
              tunnel: w786 -> [w793 _]
              frame False {
              }
              frame True {
              }
            }
            n265 = Index Array(array=w780) -> ()  [unwired: 16 in, 16 out]
            n266 = Index Array(array=w780, index=w781) -> (element=w784:dbl)
            n267 = call "Average_flow_x_time.vi"("Array of timestamps"=w788, "Previous Flow"=w787, "Latest Flow"=w784) -> ("Volume (SL)"=w790:dbl)  [unwired: 8 in]
            n268 = case shown="False" "Pause?" {
              tunnel: w789 -> [w797 w798]
              tunnel: w790 -> [w796 _]
              tunnel: [w795 w798] -> w785
              frame False {
                n269 = Add(x=w796, y=w797) -> (x+y=w795:dbl)
              }
              frame True {
              }
            }
            "Integrated Flow (SL)" <- w785
            n270 = Index Array(array=w782) -> (element #1=→"Coldhead" →"Temp A":dbl, element #2=→"Heater" →"Temp B":dbl)  [unwired: 3 in, 1 out]
            n271 = Index Array(array=w783) -> ()  [unwired: 16 in, 16 out]
            "9207 (V; A) Converted" <- w780
            "9216 #1 (°C)" <- w783
            "9216 #2 (°C)" <- w783
          }
          frame #6 {
            # "The same order applies to the headers resaved,\nbut with an additional line, stating the date/time"
            # "-----------DATA SAVED----------\nHuman-readable timestamp  ;\nTemperatures (16),  2xNI 9216;\nTemperatures (8),        NI 9226;\nVolts, Amps  (8 x2),     NI 9207;\nTemperature (2),    Lakeshore;\nHeater power (1),  Lakeshore;\nSetpoint (1),           Lakeshore;\nHV readouts (16)          CAEN ;\nCurrent time (s)                ---   ;\nCycle time (s)                    ---   ;"
            # "Saving data"
            n272 = Get Date/Time In Seconds() -> (seconds since 1Jan1904=w821:timestamp)
            n273 = To Double Precision Float(number=w821) -> (double precision float=w804:dbl)
            n274 = Build Array (concatenate)(w807, w799, w800, w801, w802, w803, w804, w805) -> (w820:dbl[])
            n275 = Array Size(array=w807) -> (size(s)=w808:i32)
            n276 = Array Size(array=w799) -> (size(s)=w809:i32)
            n277 = Add(x=w808, y=w809) -> (x+y=w806:i32)
            n278 = Get Date/Time String() -> (date string=w814:string)  [unwired: 3 in, 1 out]
            n279 = case shown="True" "Re-save headers" {
              tunnel: w806 -> [_ w822]
              frame False {
                # "Just sit around and feel pretty"
              }
              frame True {
                w830 = ""
                # "Append line of most recent channel names to header file"
                n280 = local read "Channel Names (CAEN)"() -> (w829:string[])
                n281 = local read "Channel Names (9207, ai0:7)"() -> (w837:string[])
                n282 = for {
                  N: w822 -> [_]
                  shift-right: [w861] -> w833
                  shift-left: "" -> [w862]
                  i -> [w866]
                  n283 = Format Into String(initial string="t", w866) -> (resulting string=w864:string)  [unwired: 2 in, 1 out]
                  n284 = Concatenate Strings(w862, w864, "\t") -> (w861:string)
                }
                n285 = for {
                  shift-right: [w859] -> w835
                  shift-left: w830 -> [w860]
                  tunnel: w837 -> [w857] mode=indexing
                  n286 = Concatenate Strings(w860, w857, "\t") -> (w859:string)
                }
                n287 = local read "Channel Names (9207, ai8:15)"() -> (w836:string[])
                n288 = for {
                  tunnel: w829 -> [w851] mode=indexing
                  shift-right: [w849] -> w824
                  shift-left: w830 -> [w848]
                  n289 = Concatenate Strings(w848, w851, " (V)", "\t") -> (w849:string)
                }
                n290 = for {
                  shift-right: [w855] -> w832
                  shift-left: w835 -> [w856]
                  tunnel: w836 -> [w853] mode=indexing
                  n291 = Concatenate Strings(w856, w853, "\t") -> (w855:string)
                }
                n292 = for {
                  tunnel: w829 -> [w846] mode=indexing
                  shift-right: [w844] -> w828
                  shift-left: w824 -> [w843]
                  n293 = Concatenate Strings(w843, w846, " (I)", "\t") -> (w844:string)
                }
                n294 = Get Date/Time String() -> (date string=w841:string)  [unwired: 3 in, 1 out]
                n295 = Format Date/Time String() -> (date/time string=w823:string)  [unwired: 3 in]
                n296 = Build Path(base path=path "D:/Log_data/SC_LOG_HEADERS", name or relative path=w841) -> (appended path=w840:path)
                n297 = Concatenate Strings("Time\t", w833, w832, "Temp A\tTemp B\tHeater Power\tSetpoint\t", w828, "Time in seconds\tTime per cycle\t", w823, "\r\n") -> (w825:string)
                n298 = call <vilib>:"Write Spreadsheet String.vi"("append to file? (new file:F)"=TRUE, "spreadsheet string"=w825, "file path (dialog if empty)"=w840) -> ()  [unwired: 7 in, 2 out]
              }
            }
            n299 = Build Path(base path=path "D:/Log_data/SC_LOG", name or relative path=w814) -> (appended path=w813:path)
            n300 = Format Date/Time String() -> (date/time string=w818:string)  [unwired: 3 in]
            n301 = Array To Spreadsheet String(array=w820, 3:"%.3f" ("format string")) -> (spreadsheet string=w816:string)  [unwired: 1 in]
            n302 = Concatenate Strings(w818, "\t", w816) -> (w812:string)
            n303 = call <vilib>:"Write Spreadsheet String.vi"("append to file? (new file:F)"=TRUE, "spreadsheet string"=w812, "file path (dialog if empty)"=w813) -> ()  [unwired: 7 in, 2 out]
          }
          frame #7 {
            # "Status is True if ANY (armed)\ncondition is met"
            # "Detector P. Alert"
            # "Uninteruptable\n Power Supply Alert"
            # "Temp. Warning"
            # "Arms"
            # "Comm. Alert"
            # "Temperature Alert"
            # "Alarm conditions (Temp)"
            # "Check Alarms and Warnings"
            n304 = Index Array(array=w869) -> (element #1=w868:errorcluster, element #2=w867:errorcluster)  [unwired: 2 in]
            n305 = Unbundle By Name(w913) -> ("error out.status"=w895:bool)
            "NI mod 2&3 status" <- w895
            n306 = Unbundle By Name(w926) -> ("error out.status"=w924:bool)
            "LakeShore status" <- w924
            n307 = Unbundle By Name(w925) -> ("error out.status"=w921:bool)
            "NI mod1 (P) status" <- w921
            n308 = Unbundle By Name(w867) -> ("status"=w922:bool)
            "CAEN 2 status" <- w922
            n309 = Unbundle By Name(w868) -> ("status"=w923:bool)
            "CAEN 1 status" <- w923
            n310 = Build Array(w924, w923, w922, w921, w895) -> (w896:bool[])
            n311 = Build Array("LakeShore", "CAEN 1", "CAEN 2", "NI mod 2&3", "NI mod 1") -> (w891:bool[])
            n312 = call "check_ups.vi"() -> ("Error: no voltages read"=w875:bool, "Timestamp last measured"=→"Timestamp last \nmeasured (UPS)":timestamp, "Minimum input voltage measured"=w885:dbl)  [unwired: 8 in, 1 out]
            "Minimum input voltage measured" <- w885
            n313 = property on="Det.P input #" class="DigNum (strict)"() -> ("Value"=w911:i32)  [unwired: 2 in, 2 out]
            n314 = Or Array Elements(Boolean array=w896) -> (logical OR=→"Comm. status":bool)
            n315 = for {
              tunnel: w896 -> [w929] mode=indexing
              tunnel: w891 -> [w928] mode=indexing
              tunnel: [w927] -> w890 mode=indexing
              n316 = And(x=w929, y=w928) -> (x .and. y?=w927:bool)
            }
            n317 = Index Array(array=w912, index=w911) -> (element=w908:dbl)
            n318 = Less?(x=w885, y="UPS Voltage \nLower Threshold") -> (x < y?=w877:bool)
            n319 = Equal?(x=w885, y=-1.0) -> (x = y?=w876:bool)
            n320 = Less?(x=w908, y="Underpressure threshold") -> (x < y?=w906:bool)
            n321 = Build Array(w877, w876, w875) -> (w874:bool[])
            n322 = Or Array Elements(Boolean array=w890) -> (logical OR=w880:bool)
            n323 = Greater?(x=w908, y="Overpressure threshold") -> (0:w907:bool)
            n324 = Or(x=w907, y=w906) -> (x .or. y?=w905:bool)
            "Det. P. warning" <- w905
            n325 = Or Array Elements(Boolean array=w874) -> (logical OR=w873:bool)
            "Warning" <- w873
            n326 = And(x="UPS", y=w873) -> (x .and. y?=w879:bool)
            n327 = And(x=w905, y="Detector Pressure") -> (x .and. y?=w881:bool)
            n328 = Build Array("T 1", "T 2", "T 3", "T 4", "T 5", "T 6") -> (w871:bool[])
            n329 = for {
              tunnel: w870 -> [w930] mode=indexing
              tunnel: w871 -> [w933] mode=indexing
              tunnel: [w932] -> w882 mode=indexing
              tunnel: [w931] -> w897 mode=indexing
              n330 = Less?(x=w930, y="Low Temp threshold") -> (x < y?=w935:bool)
              n331 = Greater?(x=w930, y="High Temp threshold") -> (0:w934:bool)
              n332 = Or(x=w935, y=w934) -> (x .or. y?=w931:bool)
              n333 = And(x=w933, y=w931) -> (x .and. y?=w932:bool)
            }
            n334 = Index Array(array=w897) -> (element #1=→"Boolean":bool, element #2=→"Boolean 2":bool, element #3=→"Boolean 3":bool, element #4=→"Boolean 4":bool, element #5=→"Boolean 5":bool, element #6=→"Boolean 6":bool)  [unwired: 6 in]
            n335 = Build Array (concatenate)(w882, w881, w880, w879) -> (w878:bool[])
            n336 = Or Array Elements(Boolean array=w878) -> (logical OR=w872:bool)
            "Alarm state" <- w872
          }
          frame #8 {
            # "Testing alarm will not interfere"
            # "Act on alarm"
            n337 = Or(x="Test alarm", y=w944) -> (x .or. y?=w945:bool)
            n338 = case shown="True" w945 {
              tunnel: "Test alarm" -> [_ w952]
              tunnel: w942 -> [_ w960]
              tunnel: w938 -> [_ w959]
              tunnel: w941 -> [w948 w950]
              tunnel: "Alarm\nMaster switch" -> [_ w957]
              tunnel: [w948 w951] -> w939
              frame False {
                # "Timer stays at previous value"
              }
              frame True {
                n339 = Get Date/Time In Seconds() -> (seconds since 1Jan1904=w964:timestamp)
                n340 = case shown="True" "\"Sound\" alarm" {
                  frame False {
                  }
                  frame True {
                    n341 = call <vilib>:"Beep.vi"("use system alert? (T)"=FALSE, "duration (msec)"=u32 1000, "frequency (Hz)"="Sound alarm\nFrequency (Hz)") -> ()  [unwired: 9 in]
                  }
                }
                n342 = To Double Precision Float(number=w964) -> (double precision float=w961:dbl)
                n343 = Multiply(x="Repeat Alarm SMS\nevery N minutes", y=60.0) -> (x*y=w953:dbl)
                n344 = Subtract(x=w961, y=w950) -> (x-y=w956:dbl)
                n345 = Greater?(x=w956, y=w953) -> (0:w958:bool)
                n346 = And(x=w957, y=w958) -> (x .and. y?=w955:bool)
                n347 = Or(x=w952, y=w955) -> (x .or. y?=w954:bool)
                n348 = case shown="True" w954 {
                  tunnel: w952 -> [_ w980]
                  tunnel: w960 -> [_ w988]
                  tunnel: w959 -> [_ w969]
                  tunnel: [w968 w978] -> w951
                  tunnel: w950 -> [w968 w977]
                  frame False {
                    # "Alarm not armed, or defined time has not yet passed"
                  }
                  frame True {
                    # "Average T in Det."
                    n349 = local read "Det.P input #"() -> (w993:i32)
                    n350 = case shown="True" w980 {
                      tunnel: ["Error encountered inXAMS! Status:" "TESTING the XAMS alarm. Status:"] -> w987
                      tunnel: [w997 w1000] -> w978
                      tunnel: w977 -> [_ w1000]
                      frame False {
                        n351 = Get Date/Time In Seconds() -> (seconds since 1Jan1904=w998:timestamp)
                        n352 = To Double Precision Float(number=w998) -> (double precision float=w997:dbl)
                      }
                      frame True {
                      }
                    }
                    n353 = for {
                      tunnel: w969 -> [w1002] mode=indexing
                      tunnel: [w1009] -> w972 mode=indexing
                      i -> [w1003]
                      n354 = Format Into String(format string="%.0f", w1003) -> (resulting string=w1007:string)  [unwired: 2 in, 1 out]
                      n355 = Format Into String(format string="%.1f", w1002) -> (resulting string=w1005:string)  [unwired: 2 in, 1 out]
                      n356 = Concatenate Strings("\n" ("format string"), w1007, "     " ("format string"), w1005) -> (w1009:string)
                    }
                    n357 = Index Array(array=w988, index=w993) -> (element=w989:dbl)
                    n358 = Array Size(array=w969) -> (size(s)=w991:i32)
                    n359 = Add Array Elements(numeric array=w969) -> (sum=w992:dbl)
                    n360 = Format Into String(format string="%.3f", w989) -> (resulting string=w983:string)  [unwired: 2 in, 1 out]
                    n361 = Divide(x=w992, y=w991) -> (x/y=w981:dbl)
                    n362 = Format Date/Time String() -> (date/time string=w985:string)  [unwired: 3 in]
                    n363 = Format Into String(format string="%.2f", w981) -> (resulting string=w970:string)  [unwired: 2 in, 1 out]
                    n364 = Concatenate Strings(w987, "\nDate/time: ", w985, "\nDetector Pressure: ", w983, " bar", "\nDetector Temperatures (°C):", "\nCh:   Temp:" ("format string"), w972, "\nAverage detector temperature: ", w970) -> (w976:string)
                    "Alarm (or test) message" <- w976
                    n365 = for {
                      tunnel: w976 -> [w996]
                      tunnel: "Phone numbers" -> [w995] mode=indexing
                      n366 = call "send_sms.vi"("Message content"=w996, "Phone number"=w995) -> ("standard error"=→"SMS error":string)  [unwired: 8 in, 1 out]
                    }
                  }
                }
              }
            }
            n367 = And(x="Shut off heater \nif Alarm is active", y=w944) -> (x .and. y?=w946:bool)
            "Alarm active 2" <- "Alarm\nMaster switch"
          }
          frame #9 {
            # "Daily e-mail"
            n368 = Get Date/Time In Seconds() -> (seconds since 1Jan1904=w1024:timestamp)
            n369 = To Double Precision Float(number=w1024) -> (double precision float=w1023:dbl)
            n370 = Get Date/Time String(want seconds? (F)=FALSE) -> (time string=w1026:string)  [unwired: 2 in, 1 out]
            n371 = Subtract(x=w1023, y=w1016) -> (x-y=w1022:dbl)
            n372 = Equal?(x=w1026, y="Send status email at time:") -> (x = y?=w1019:bool)
            n373 = Greater?(x=w1022, y=62) -> (0:w1018:bool)
            n374 = Build Array("Send daily email?", w1019, w1018) -> (w1017:bool[])
            n375 = And Array Elements(Boolean array=w1017) -> (logical AND=w1013:bool)
            n376 = Or(x="Send status email now", y=w1013) -> (x .or. y?=w1014:bool)
            n377 = case shown="True" w1014 {
              tunnel: w1011 -> [_ w1031]
              tunnel: w1029 -> [_ w1048]
              tunnel: w1028 -> [_ w1057]
              tunnel: w1016 -> [w1030 _]
              tunnel: [w1030 w1043] -> w1015
              frame False {
              }
              frame True {
                # "Average T in Det."
                n378 = Not Equal To 0?(x="Number of Bonus lines") -> (x != 0?=w1036:bool)
                n379 = case shown="True" w1036 {
                  tunnel: [w1068 w1071] -> w1037
                  tunnel: "Number of Bonus lines" -> [_ w1074]
                  frame False {
                    n380 = Build Array("\n[Flavor text module inactive]") -> (w1068:string[])
                  }
                  frame True {
                    n381 = Build Path(base path=path "C:/Users/xams/Desktop/New XAMS Slow Control", name or relative path="cool_beans.txt") -> (appended path=w1075:path)
                    n382 = call-poly <vilib>:"Read Delimited Spreadsheet.vi"("file path (dialog if empty)"=w1075) -> ("all rows"=w1078:string[][])  [unwired: 9 in, 5 out]
                    n383 = Array Size(array=w1078) -> (size(s)=w1080:i32[])
                    n384 = Index Array(array=w1080) -> (element=w1079:i32)  [unwired: 1 in]
                    n385 = for {
                      N: w1074 -> [_]
                      tunnel: w1079 -> [w1085]
                      tunnel: w1078 -> [w1084]
                      tunnel: [w1081] -> w1072 mode=indexing
                      n386 = Random Number (0-1)() -> (number: 0 to 1=w1088:dbl)
                      n387 = Multiply(x=w1085, y=w1088) -> (x*y=w1087:dbl)
                      n388 = Round To Nearest(number=w1087) -> (nearest integer value=w1086:dbl)
                      n389 = Index Array(array=w1084, index (row)=w1086) -> (element=w1082:string[])  [unwired: 1 in]
                      n390 = Concatenate Strings("\n", w1082) -> (w1081:string)
                    }
                    n391 = Concatenate Strings("\n\nCool beans of the day: ", w1072) -> (w1070:string)
                    n392 = Build Array(w1070) -> (w1071:string[])
                  }
                }
                n393 = local read "Det.P input #"() -> (w1058:i32)
                n394 = for {
                  tunnel: [w1097] -> w1050 mode=indexing
                  tunnel: w1031 -> [w1089] mode=indexing
                  i -> [w1090]
                  n395 = Format Into String(format string="%.0f", w1090) -> (resulting string=w1094:string)  [unwired: 2 in, 1 out]
                  n396 = Format Into String(format string="%.2f", w1089) -> (resulting string=w1092:string)  [unwired: 2 in, 1 out]
                  n397 = Concatenate Strings("\nCh: " ("format string"), w1094, ", Temp: " ("format string"), w1092, "°C." ("format string")) -> (w1097:string)
                }
                n398 = Array Size(array=w1031) -> (size(s)=w1066:i32)
                n399 = Add Array Elements(numeric array=w1031) -> (sum=w1067:dbl)
                n400 = Index Array(array=w1057, index=w1058) -> (element=w1055:dbl)
                n401 = Divide(x=w1067, y=w1066) -> (x/y=w1064:dbl)
                n402 = Format Into String(format string="%.3f", w1055) -> (resulting string=w1053:string)  [unwired: 2 in, 1 out]
                n403 = Format Into String(format string="%.2f", w1064) -> (resulting string=w1047:string)  [unwired: 2 in, 1 out]
                n404 = Select(t="ACTIVE!!!!!", s=w1048, f="inactive.") -> (s? t:f=w1060:string)
                n405 = Concatenate Strings("Hello, XAMS teammembers.", "\n\nThe alarm is currently ", w1060, "\n\nThe latest detector pressure is: ", w1053, " bar." ("format string"), "\nTemperatures inside the detector are:", w1050, "\nThe average detector temperature is ", w1047, "°C." ("format string"), "\n\nThank you for doing your best today, once again!\nRegards, SC.", w1037) -> (w1042:string)
                "Status email preview" <- w1042
                n406 = call "custom_email_program.vi"("mail server"="smtp.nikhef.nl", "return address"="return address", "message"=w1042, "subject ([No Subject])"="XAMS daily status email.", "Email Adresses"="Email Addresses") -> ("error out"=w1034:errorcluster)  [unwired: 6 in]
                n407 = Unbundle By Name(w1034) -> ("code"=→"Email error":i32, "source"=→"source":string)
                n408 = Get Date/Time In Seconds() -> (seconds since 1Jan1904=w1044:timestamp)
                n409 = To Double Precision Float(number=w1044) -> (double precision float=w1043:dbl)
              }
            }
          }
        }
        n410 = Decrement(x="Cycles to execute") -> (x-1=w288:dbl)
        n411 = Decrement(x=w288) -> (x-1=w287:dbl)
        n412 = Greater?(x=w271, y=w287) -> ()  [unwired: 1 out]
        n413 = Decrement(x="Clear data every N cycles") -> (x-1=w268:dbl)
        n414 = Greater?(x=w271, y=w268) -> (0:w270:bool)
        n415 = And(x="Auto-clear data?", y=w270) -> (x .and. y?=w273:bool)
        n416 = Or(x=w273, y="Clear data") -> (x .or. y?=w275:bool)
        n417 = case shown="False" w275 {
          tunnel: w286 -> [w314 _]
          tunnel: [w314 dbl[][] []] -> w285
          tunnel: w284 -> [w313 _]
          tunnel: [w313 w320] -> w283
          tunnel: w282 -> [w312 _]
          tunnel: [w312 w320] -> w281
          tunnel: w280 -> [w311 _]
          tunnel: [w311 w318] -> w279
          tunnel: w278 -> [w310 _]
          tunnel: [w310 w316] -> w277
          tunnel: w271 -> [w309 _]
          tunnel: [w309 0] -> w272
          frame False {
          }
          frame True {
            w320 = 0.0
            n418 = Get Date/Time In Seconds() -> (seconds since 1Jan1904=w317:timestamp)
            n419 = To Double Precision Float(number=w317) -> (double precision float=w319:dbl)
            n420 = Build Array(w317) -> (w316:timestamp[])
            n421 = Build Array(w319, w319) -> (w318:dbl[])
          }
        }
        n422 = Or(x=FALSE, y="stop") -> (x .or. y?=w306:bool)
        "Auto-clear" <- "Auto-clear data?"
      }
    }
    frame True {
    }
  }
  n423 = Array Size(array=w30) -> (size(s)=w33:i32)
  n424 = Decrement(x=w33) -> (x-1=w32:i32)
  n425 = Index Array(array=w30, index #1=w32, index #2=1 ("index")) -> (element #1=w31:timestamp, element #2=w16:timestamp)
  n426 = To Double Precision Float(number=w31) -> (double precision float=w29:dbl)
  n427 = To Double Precision Float(number=w16) -> (double precision float=w28:dbl)
  n428 = flat-sequence {
    tunnel: w23 -> [w1142]
    tunnel: w19 -> [w1114]
    tunnel: w18 -> [w1132]
    tunnel: w11 -> [w1121]
    tunnel: w6 -> [w1118]
    tunnel: w1 -> [w1112]
    frame #0 {
      w1138 = u16 2 items=["1"=1, "2"=2] ("Heater Output (1:1)")
      w1139 = u16 0 items=["Off", "Low (On)", "Medium", "High"] ("Range (0:Off)")
      # "The voltages over the components do NOT get reset by these icons,\nonly the communication gets stopped and references closed."
      # "Important icons! Always press STOP button when done \ninstead of force closing, otherwise these don't get executed"
      # "Turn off heater, shutdown COM"
      # "Error Handling and Post-Processing (EHaPP)"
      n429 = Unbundle(w1142) -> ("VISA resource name out"=w1141:refnum<visa-resource-name>, "error out"=w1140:errorcluster)
      n430 = Unbundle(w1132) -> ("task out"=w1130:refnum<k21>, "error out"=w1128:errorcluster)
      n431 = Unbundle(w1121) -> ("task out"=w1125:refnum<k21>, "error out"=w1123:errorcluster)
      n432 = Unbundle(w1118) -> ("task out"=w1117:refnum<k21>, "error out"=w1116:errorcluster)
      n433 = Index Array(array=w1114) -> (element=w1113:T4)  [unwired: 1 in]
      n434 = Index Array(array=w1112) -> (element #1=w1110:errorcluster, element #2=w1109:errorcluster)  [unwired: 2 in]
      n435 = Merge Errors(w1110, w1109) -> (w1108:errorcluster)
      n436 = Unbundle(w1113) -> ("VISA resource name"=w1133:refnum<visa-resource-name>)  [unwired: 2 out]
      n437 = call <vilib>:"DAQmx Stop Task.vi"("task/channels in"=w1130, "error in"=w1128) -> ("task out"=w1129:refnum<k21>, "error out"=w1127:errorcluster)  [unwired: 12 in]
      n438 = call <vilib>:"DAQmx Stop Task.vi"("task/channels in"=w1125, "error in"=w1123) -> ("task out"=w1124:refnum<k21>, "error out"=w1122:errorcluster)  [unwired: 12 in]
      n439 = call <vilib>:"DAQmx Stop Task.vi"("task/channels in"=w1117, "error in"=w1116) -> ("task out"=w1115:refnum<k21>, "error out"=w1119:errorcluster)  [unwired: 12 in]
      n440 = call <instrlib>:"Configure Output Range and Manual Value.vi"("VISA resource name"=w1141, "Heater Output (1:1)"=w1138, "Range (0:Off)"=w1139, "Manual Output (0.00 %)"=0.0, "error in (no error)"=w1140) -> ("VISA resource name out"=w1136:refnum<visa-resource-name>, "error out"=w1135:errorcluster)  [unwired: 9 in]
      n441 = call <instrlib>:"Close.vi"("error in (no error)"=w1108, "VISA resource name"=w1133) -> ("error out"=w1111:errorcluster)  [unwired: 9 in]
      n442 = call <instrlib>:"Close.vi"("error in (no error)"=w1135, "VISA resource name"=w1136) -> ("error out"=w1134:errorcluster)  [unwired: 9 in]
      n443 = call <vilib>:"DAQmx Clear Task.vi"("task in"=w1129, "error in"=w1127) -> ("error out"=w1131:errorcluster)  [unwired: 13 in]
      n444 = call <vilib>:"DAQmx Clear Task.vi"("task in"=w1124, "error in"=w1122) -> ("error out"=w1126:errorcluster)  [unwired: 13 in]
      n445 = call <vilib>:"DAQmx Clear Task.vi"("task in"=w1115, "error in"=w1119) -> ("error out"=w1120:errorcluster)  [unwired: 13 in]
      n446 = Merge Errors(w1111, w1108) -> (w1107:errorcluster)
      n447 = call <vilib>:"Simple Error Handler.vi"("error in (no error)"=w1134) -> ()  [unwired: 4 in, 5 out]
      n448 = call <vilib>:"Simple Error Handler.vi"("error in (no error)"=w1131) -> ()  [unwired: 4 in, 5 out]
      n449 = call <vilib>:"Simple Error Handler.vi"("error in (no error)"=w1126) -> ()  [unwired: 4 in, 5 out]
      n450 = call <vilib>:"Simple Error Handler.vi"("error in (no error)"=w1120) -> ()  [unwired: 4 in, 5 out]
      n451 = call <vilib>:"Simple Error Handler.vi"("error in (no error)"=w1107) -> ()  [unwired: 4 in, 5 out]
    }
  }
  n452 = Subtract(x=w29, y=w28) -> ()  [unwired: 1 out]
  "Started up?" <- w27
